vi "lightsheetMain.vi"() -> ()   [LabVIEW 2015]
panel:
  out "initLasers":T1(array[cluster])=[{"Component ID"="405nm", "COM Port"="COM14", "Type "=enum."omicronLuxX", "init"=1, "Max power (mW)"=60.0}, {"Component ID"="488nm", "COM Port"="COM4", "Type "=enum."omicronLuxX", "init"=1, "Max power (mW)"=60.0}, {"Component ID"="561nm", "COM Port"="COM27", "Type "=enum."coherentObis", "init"=1, "Max power (mW)"=50.0}, {"Component ID"="642nm", "COM Port"="COM12", "Type "=enum."omicronLuxX", "init"=1, "Max power (mW)"=140.0}]
  out "acquisitionTime":u32
  out "opticalSectionThickness (um)":dbl=5.0
  out "acqLaserCOM":refnum<visa-resource-name>[](array[refnum])
  out "acqLaserOff":string[](array[string])
  out "acqLaserOn":string[](array[string])
  out "acqFW":u8[](array[numeric])
  out "Lat x inc (mm)":dbl=0.37273599999999996
  out "Lat y inc (mm)":dbl=0.37273599999999996
  out "no y steps":i32=1
  out "no colours":i32=1
  out "no z imgs (acq)":i32=1
  out "no x steps":i32=1
  out "stop live view":bool
  out "LH yLim (mm)":dbl
  out "RH yLim (mm)":dbl
  in  "Set RH yLim":bool
  in  "Set LH yLim":bool
  out "TH zLim (mm)":dbl
  in  "Set TH zLim":bool
  in  "acqLSFM_3":enum32{"Acquisition (hardware)"}(tab)
  out "Generating tiff stacks":bool
  out "Acquisition in progress":bool
  in  "convertDcimgToTifStacks":bool=TRUE
  in  "setupAcq":bool
  in  "testAcq":bool
  out "x1":dbl
  out "y1":dbl
  out "z1":dbl
  out "x2":dbl
  out "y2":dbl
  out "z2":dbl
  in  "no z steps":i32=1
  in  "% FOV overlap":i32=10
  in  "z inc (um)":dbl=1.0
  in  "642":bool=TRUE
  in  "561":bool=TRUE
  in  "405":bool=TRUE
  in  "488":bool=TRUE
  in  "beginAcq":bool
  in  "stopAcq":bool
  in  "end all comms and exit":bool
  in  "acquisitionMode":enum32{"stop/start  ", "cont."}(radio)
  out "z inc (mm)":dbl=0.01
  in  "Save acq vals":bool
  in  "Read acq vals":bool
  out "Filter wheel":cluster{"FW Handle":u32, "init?":i16}={"FW Handle"=428794912, "init?"=1}
  out "sCMOS":cluster{"init":i16, "sCMOS handle":u32}
  out "Z stage":T2={"System no."=2, "zIdx"=1, "zLim (mm)"=0.0, "0, 1"=0}
  out "XY stage":T3={"System no."=1, "xIdx"=1, "yIdx"=2, "xLim (mm)"=0.0, "yLim (mm)"=0.0, "0, 1"=0}
  in  "LSFM_3":T4(tab)=enum."lasers/filters"
  out "acqDelay (ms)":u32=10
  out "fine axial vel (mm/s)":dbl=10.0
  in  "set axial vel":bool
  in  "filename":string="testImg"
  in  "Index":i32
  in  "Down":bool
  in  "Up":bool
  in  "Left":bool
  in  "Right":bool
  in  "Backward":bool
  in  "Forward":bool
  in  "Axial stepsize (mm/um)":dbl=1.0
  in  "Lateral stepsize (mm/um)":dbl=1.0
  in  "Toggle coarse/fine":enum32{"Coarse (mm) ", "Fine (um) "}(radio)
  out "x (mm)":dbl
  out "y (mm)":dbl
  out "z (mm)":dbl
  in  "Snap img":bool
  in  "set init xy pos":bool
  in  "set fin xy pos":bool
  in  "set init z":bool
  in  "set fin z":bool
  in  "mov init xy":bool
  in  "mov init z":bool
  in  "mov fin xy":bool
  in  "mov fin z":bool
  in  "coarse axial vel (mm/s)":dbl=6.0
  in  "642 nm power (mW)":dbl(slide)=54.0 min=0.0 max=60.0 step=1.0 scale=0.0..140.0
  in  "561 nm power (mW)":dbl(slide)=8.0 min=0.0 max=60.0 step=1.0 scale=0.0..60.0
  in  "488 nm power (mW)":dbl(slide)=5.0 min=0.0 max=60.0 step=1.0 scale=0.0..60.0
  in  "405 nm power (mW)":dbl(slide)=5.0 min=0.0 max=60.0 step=1.0 scale=0.0..60.0
  in  "FW pos":u16(ring)=4 items=["460/36 [DAPI]"=1, "525/50 [FITC]"=2, "605/70 [Cy3]"=3, "665/LP [Cy5]"=4, "Empty-1"=5, "Empty-2"=6]
  in  "next":bool
  in  "prev":bool
  in  "642 nm ON":bool
  in  "642 nm OFF":bool
  in  "561 nm ON":bool
  in  "561 nm OFF":bool
  in  "488 nm ON":bool
  in  "488 nm OFF":bool
  in  "405 nm ON":bool
  in  "405 nm OFF":bool
  in  "405 filter":u8(ring)=1 items=["460/36 [DAPI]"=1, "525/50 [FITC]"=2, "605/70 [Cy3]"=3, "665/LP [Cy5]"=4, "Empty-1"=5, "Empty-2"=6]
  in  "488 filter":u8(ring)=2 items=["460/36 [DAPI]"=1, "525/50 [FITC]"=2, "605/70 [Cy3]"=3, "665/LP [Cy5]"=4, "Empty-1"=5, "Empty-2"=6]
  in  "561 filter":u8(ring)=3 items=["460/36 [DAPI]"=1, "525/50 [FITC]"=2, "605/70 [Cy3]"=3, "665/LP [Cy5]"=4, "Empty-1"=5, "Empty-2"=6]
  in  "642 filter":u8(ring)=4 items=["460/36 [DAPI]"=1, "525/50 [FITC]"=2, "605/70 [Cy3]"=3, "665/LP [Cy5]"=4, "Empty-1"=5, "Empty-2"=6]
  out "Acquiring?":bool
  in  "live stream":bool
  in  "Set exp. time":bool
  in  "Exposure time (s)":dbl=1.0
  in  "stop live stream":bool
  in  "View stream":bool=TRUE
  out "Img. pixel size":dbl=0.26
  out "No. of pix":u16=2048
  in  "pixel binning":u16(ring) items=["1x1"=1, "2x2"=2, "4x4"=4]
  in  "No. pix":u16=2048
  in  "scmos pixel size (um)":dbl=6.5 format="%#_13g"
  out "FOV (mm)":dbl=0.53248
  in  "sensorSize":dbl=13.312 format="%#_13g"
  in  "Mag":dbl=25.0 format="%#_13g"
  in  "z":bool
  in  "xy":bool
  in  "488nm":bool=TRUE
  in  "405nm":bool=TRUE
  in  "561nm":bool=TRUE
  in  "642nm":bool=TRUE
  in  "sCMOS":bool
  in  "FW":bool=TRUE
  out "Appended path":path=path "C:/Users/LSFM_2/Desktop/dataAcq_2705/bothIllAxis/4umBead0.tif"
  in  "Base path":path=path "C:/Users/sims01/Desktop/dataAcq"
  in  "dcimgToStack":bool
  in  "stageAccDelay (ms)":u32
  # "Stage limits"
  # "Positions"
  # "Step sizes"
  # "Currrent positions"
  # "Motion control"
  # "Move stages"
  # "lasers"
  # "filters"
  # "File setup"
  # "Hardware initialization"
  # "Microscope properties"
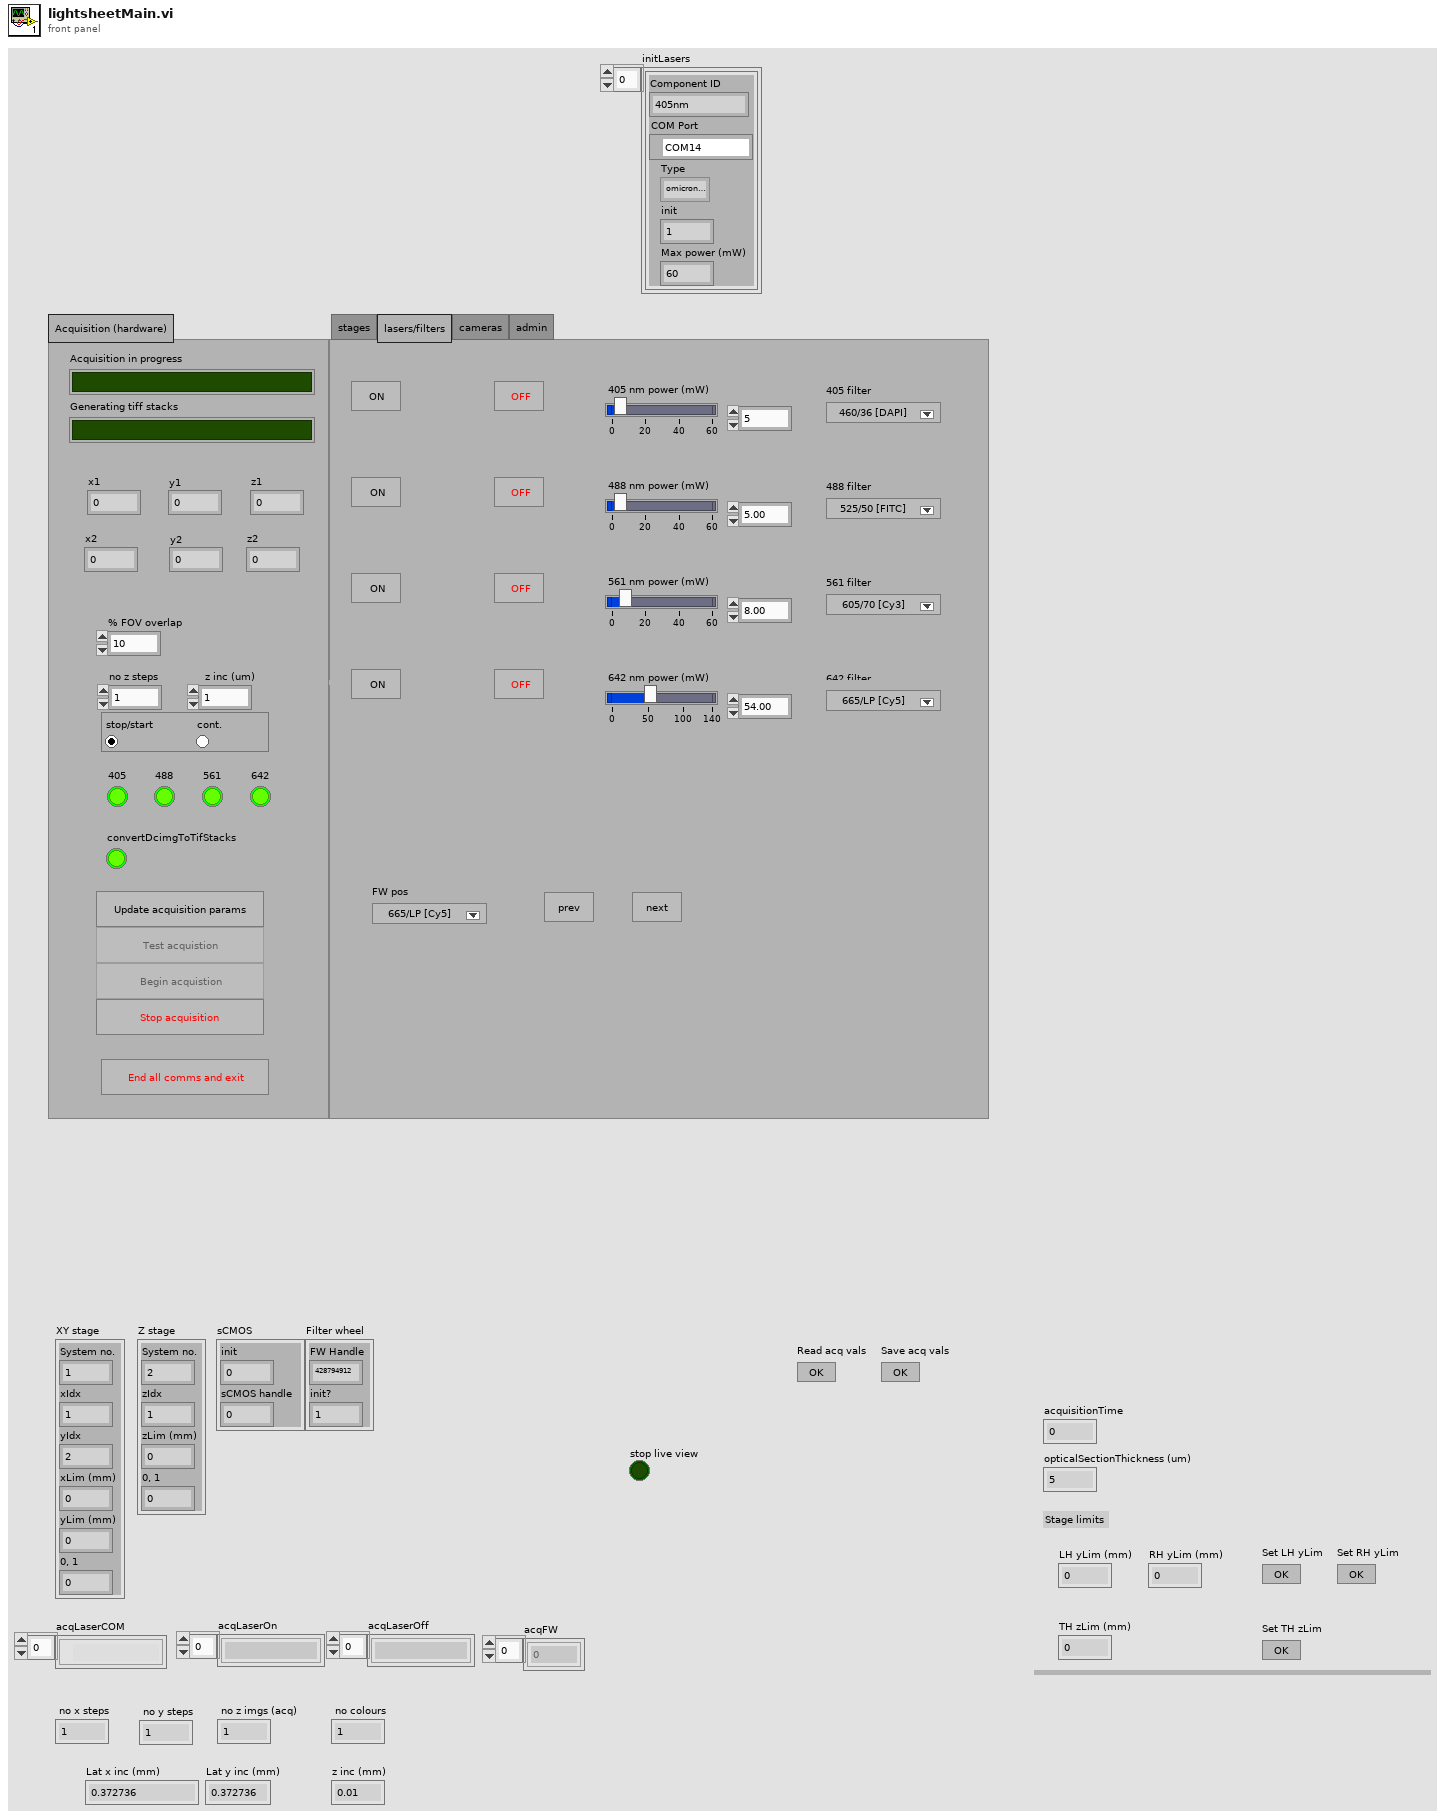
[diagram p1: front panel]
types:
  T1 = cluster{"Component ID":string, "COM Port":refnum<visa-resource-name>, "Type ":enum16{"omicronLuxX", "coherentObis"}, "init":i16, "Max power (mW)":dbl}[]
  T2 = cluster{"System no.":i32, "zIdx":i32, "zLim (mm)":dbl, "0, 1":i16}
  T3 = cluster{"System no.":i32, "xIdx":i32, "yIdx":i32, "xLim (mm)":dbl, "yLim (mm)":dbl, "0, 1":i16}
  T4 = enum32{"stages", "lasers/filters", "cameras", "admin"}
  T5 = enum8{"Enabled", "Disabled", "Disabled and Grayed Out"}
  T6 = cluster{"Component ID":string, "COM Port":refnum<visa-resource-name>, "Type ":enum16{"omicronLuxX", "coherentObis"}, "init":i16, "Max power (mW)":dbl}
  T7 = enum32{"Invalid", "Standard", "Closed", "Hidden", "Minimized", "Maximized"}
  T8 = cluster{"height":u32, "width":u32, "datatype":u32}
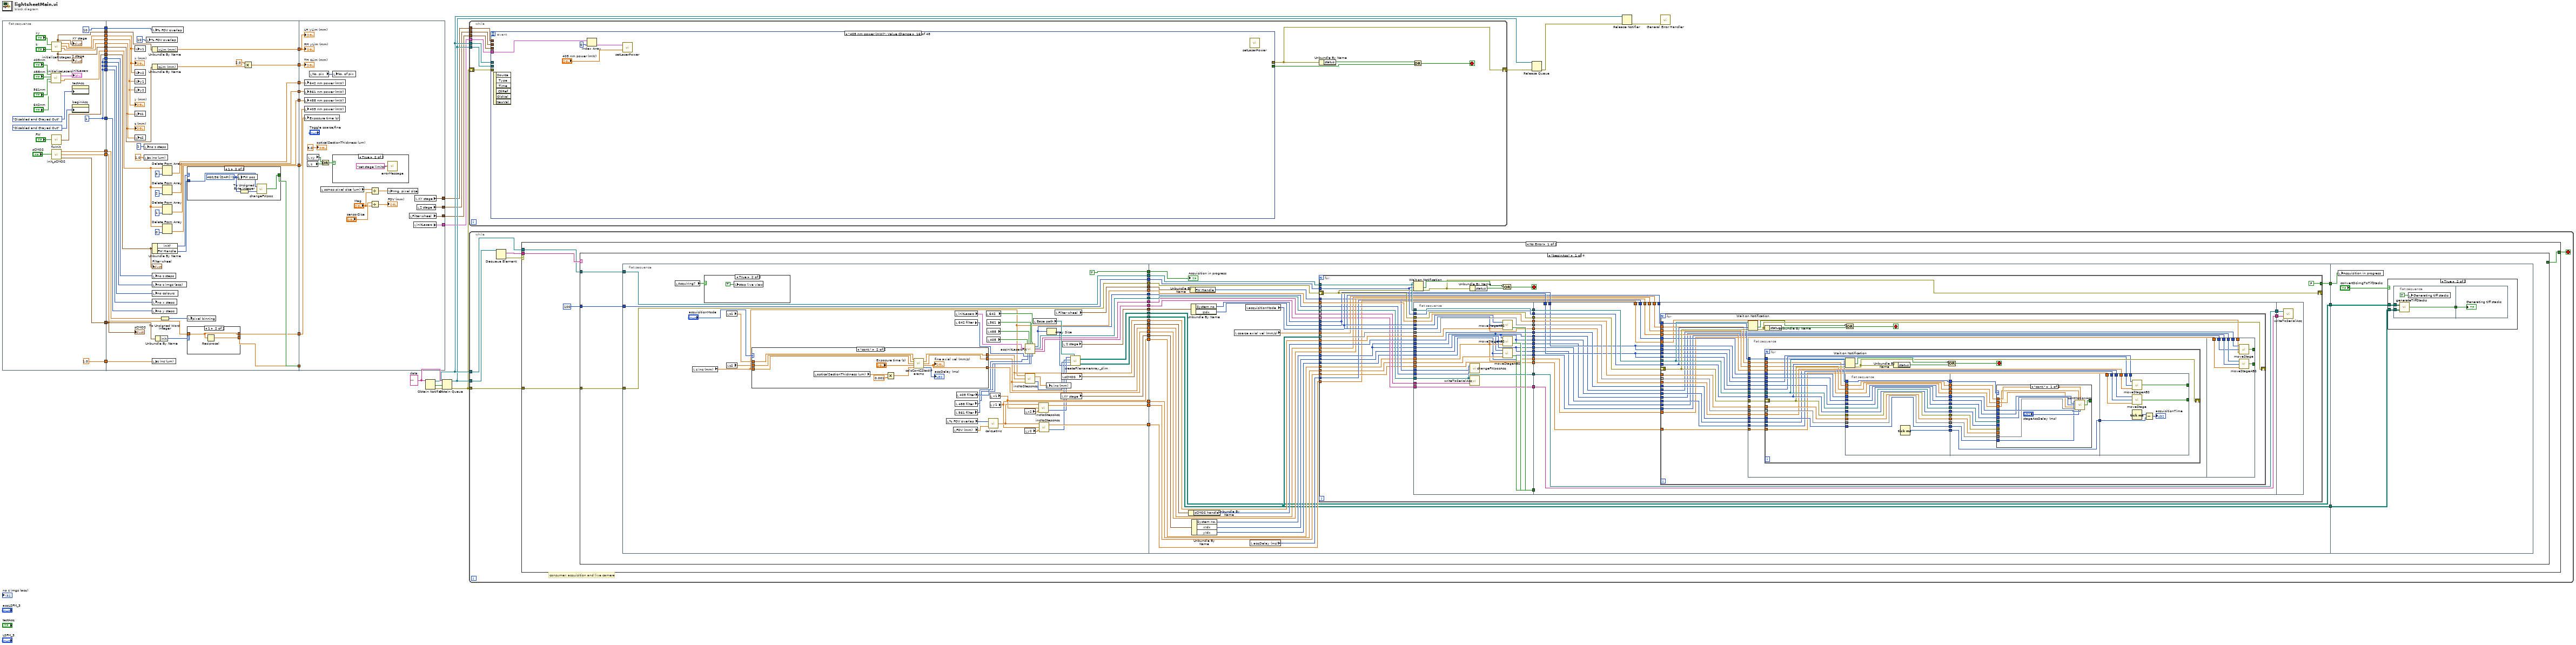
[diagram p0: block diagram]
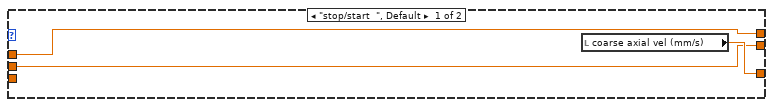
[diagram p3: hidden frame]
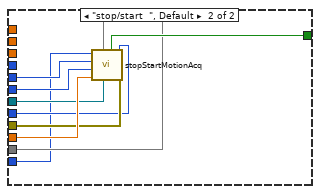
[diagram p4: hidden frame]
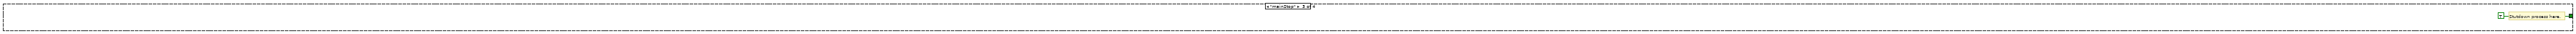
[diagram p7: hidden frame]
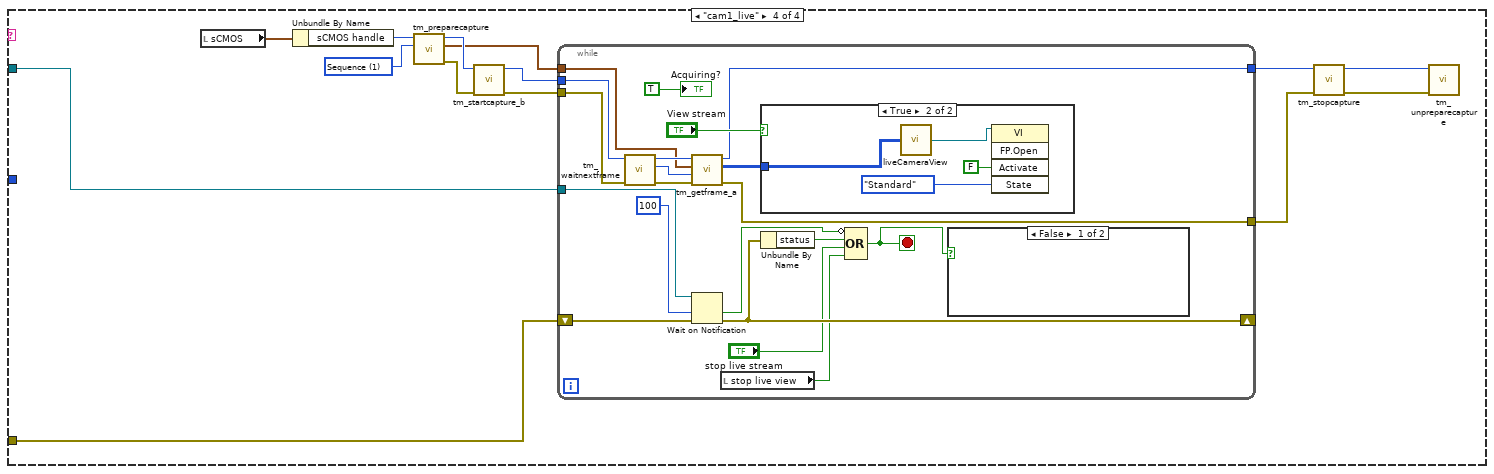
[diagram p8: hidden frame]
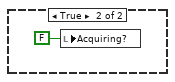
[diagram p9: hidden frame]
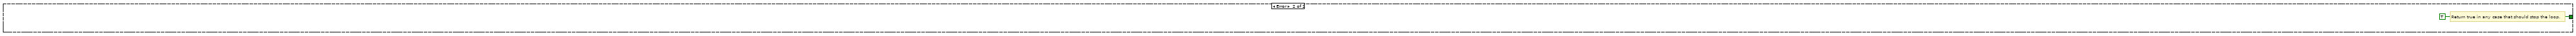
[diagram p11: hidden frame]
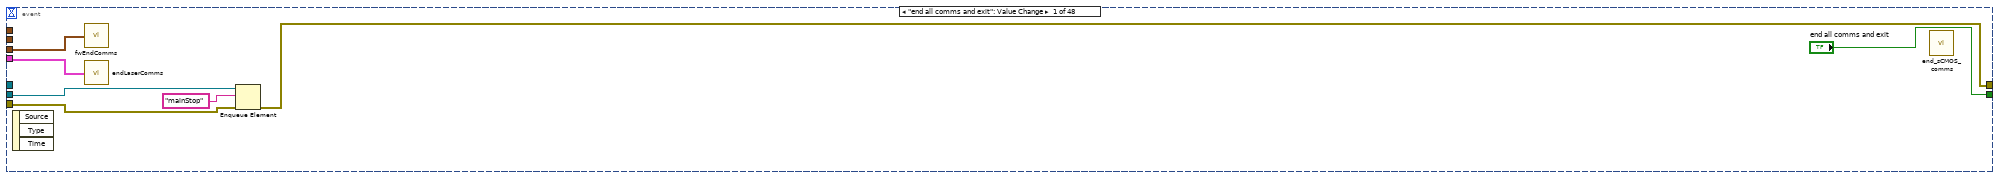
[diagram p12: hidden frame]
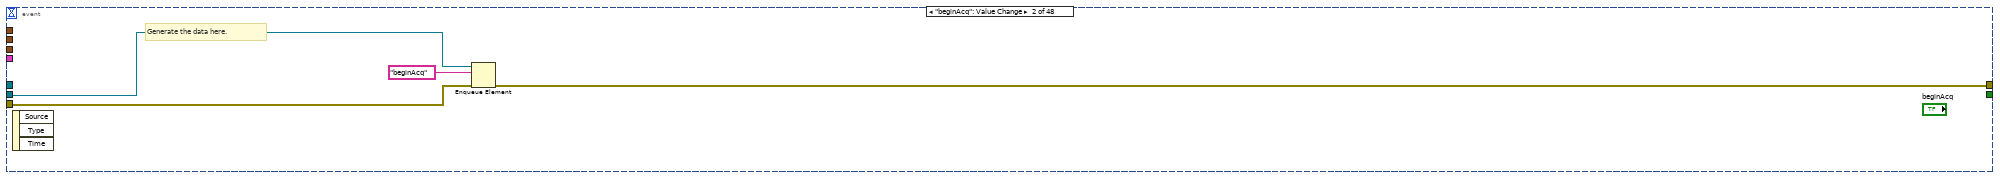
[diagram p13: hidden frame]
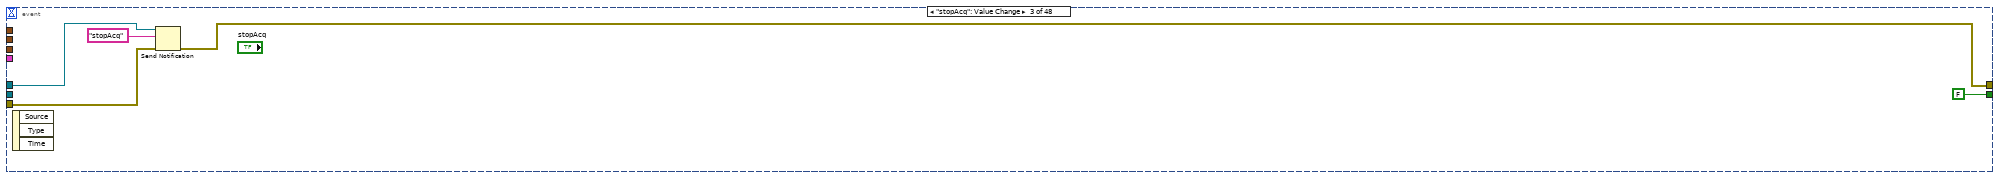
[diagram p14: hidden frame]
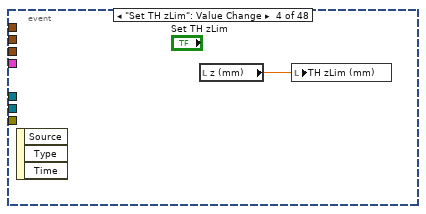
[diagram p15: hidden frame]
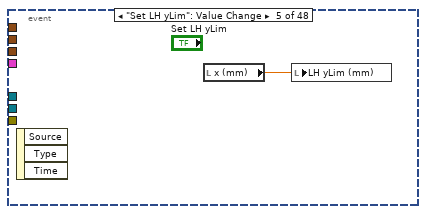
[diagram p16: hidden frame]
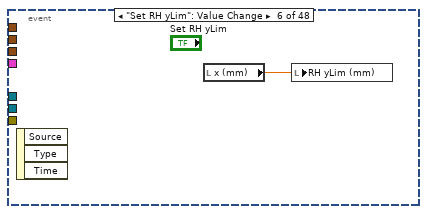
[diagram p17: hidden frame]
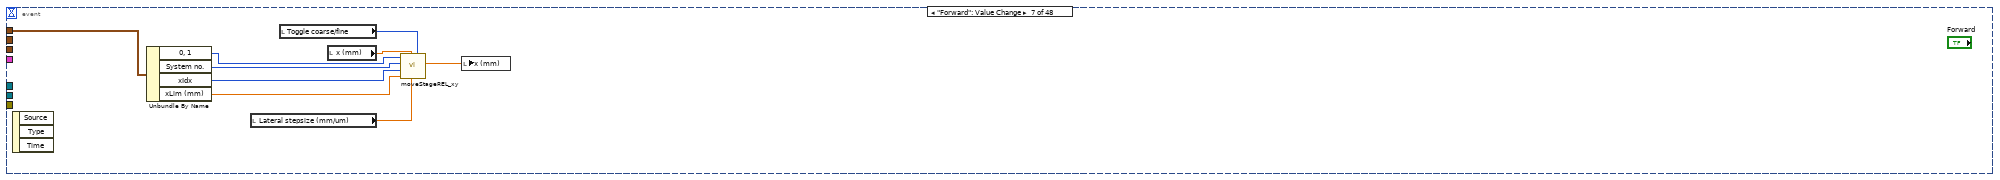
[diagram p18: hidden frame]
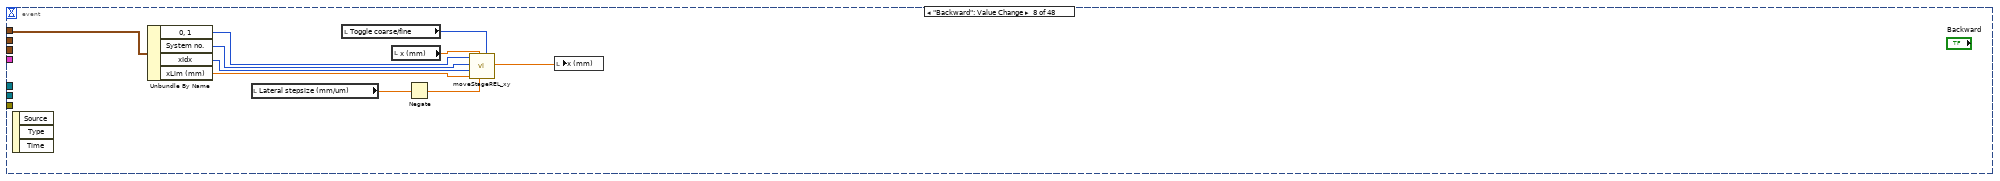
[diagram p19: hidden frame]
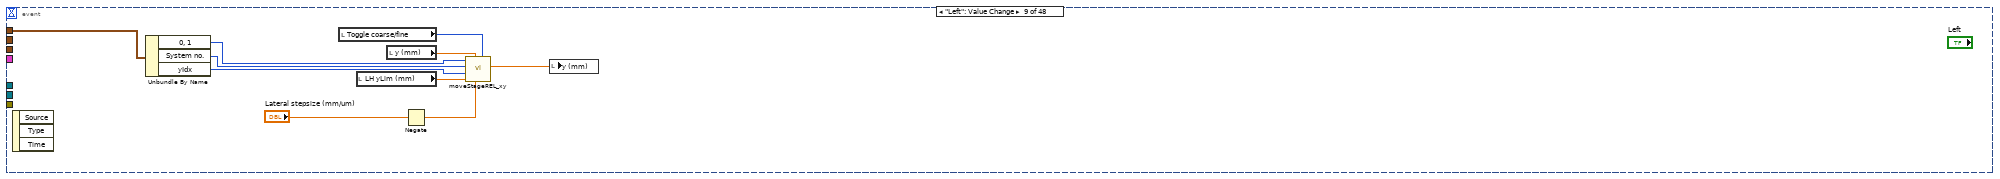
[diagram p20: hidden frame]
diagram:
  w28 = ""  # data
  n1 = flat-sequence {
    tunnel: [w61] -> w39
    tunnel: [w60] -> w38
    tunnel: [w59] -> w37
    tunnel: [w52] -> w36
    tunnel: [w51] -> w35
    tunnel: [w58] -> w34
    tunnel: [w57] -> w18
    tunnel: [w56] -> w17
    tunnel: [w50] -> w13
    tunnel: [w48] -> w12
    tunnel: [w48] -> w11
    tunnel: [w48] -> w10
    tunnel: [w48] -> w9
    tunnel: [10 ("% FOV overlap")] -> w8
    tunnel: [w48] -> w7
    tunnel: [1.0 ("z inc (um)")] -> w6
    tunnel: [w40] -> w5
    tunnel: w39 -> [w85]
    tunnel: w38 -> [w86]
    tunnel: w37 -> [w87]
    tunnel: w36 -> [w100]
    tunnel: w35 -> [w102]
    tunnel: w34 -> [w99]
    tunnel: [w96] -> w33
    tunnel: [w95] -> w32
    tunnel: [w94] -> w31
    tunnel: w18 -> [w93]
    tunnel: w17 -> [w92]
    tunnel: [w91] -> w16
    tunnel: [w90] -> w15
    tunnel: w13 -> [w81]
    tunnel: w12 -> [w80]
    tunnel: w11 -> [w79]
    tunnel: w10 -> [w78]
    tunnel: w9 -> [w77]
    tunnel: w8 -> [w76]
    tunnel: w7 -> [w75]
    tunnel: w6 -> [w74]
    tunnel: w5 -> [w65]
    tunnel: [w71] -> w4
    tunnel: [w69] -> w3
    tunnel: [w67] -> w2
    tunnel: [w64] -> w1
    tunnel: w33 -> [_]
    tunnel: w32 -> [w126]
    tunnel: w31 -> [_]
    tunnel: [w125] -> w20
    tunnel: [w124] -> w19
    tunnel: [w123] -> w21
    tunnel: w16 -> [w122]
    tunnel: w15 -> [w121]
    tunnel: [w115] -> w14
    tunnel: w4 -> [w114]
    tunnel: w3 -> [w113]
    tunnel: w2 -> [w112]
    tunnel: w1 -> [w111]
    frame #0 {
      w48 = 1 ("no y steps")
      n2 = call "initialiseLasers.vi"("642 nm"="642nm", "561 nm"="561nm", "488 nm"="488nm", "405 nm"="405nm") -> ("currLaserPowers"=w40:dbl[], "outputLasers"=→"initLasers":T1)
      n3 = call "fwInit.vi"("FW init?"="FW") -> ("Filter wheel init"=w58:cluster{"FW Handle":u32, "init?":i16})
      n4 = call "initializePIstages.vi"("xy stage"="xy", "z stage"="z") -> ("XY stage"=w56:T3, "Z stage"=w57:T2, "current xPos (mm)"=w61:dbl, "current yPos (mm)"=w60:dbl, "current zPos (mm)"=w59:dbl)  [unwired: 1 in]
      "XY stage" <- w56
      "Z stage" <- w57
      n5 = call "init_sCMOS.vi"("sCMOS_1"="sCMOS") -> ("Binning"=w50:dbl, "Exposure"=w52:dbl, "sCMOS init"=w51:cluster{"init":i16, "sCMOS handle":u32})
      n6 = property on="testAcq" class="Bool"("DisabledEnum"=T5."Disabled and Grayed Out" ("Disabled")) -> ()  [unwired: 2 in, 2 out]
      n7 = property on="beginAcq" class="Bool"("DisabledEnum"=T5."Disabled and Grayed Out" ("Disabled")) -> ()  [unwired: 2 in, 2 out]
    }
    frame #1 {
      n8 = local write "x1"(w85) -> ()
      n9 = local write "x2"(w85) -> ()
      n10 = local write "y1"(w86) -> ()
      n11 = local write "y2"(w86) -> ()
      n12 = local write "z1"(w87) -> ()
      n13 = local write "z2"(w87) -> ()
      n14 = local write "no z steps"(1 ("no z steps")) -> ()
      n15 = local write "z inc (um)"(1.0 ("z inc (um)")) -> ()
      n16 = local write "% FOV overlap"(10 ("% FOV overlap")) -> ()
      n17 = local write "% FOV overlap"(w76) -> ()
      n18 = Unbundle By Name(w92) -> ("xLim (mm)"=w91:dbl)
      n19 = Unbundle By Name(w93) -> ("zLim (mm)"=w89:dbl)
      n20 = Unbundle By Name(w99) -> ("init?"=w98:i16, "FW Handle"=w97:u32)
      n21 = local write "no z steps"(w75) -> ()
      n22 = local write "no z imgs (acq)"(w78) -> ()
      n23 = local write "no colours"(w79) -> ()
      n24 = local write "no x steps"(w77) -> ()
      n25 = local write "no y steps"(w80) -> ()
      n26 = local write "z inc (um)"(w74) -> ()
      n27 = Unbundle By Name(w102) -> ("init"=w101:i16)
      n28 = To Unsigned Word Integer(number=w81) -> (unsigned 16bit integer=w82:u16)
      n29 = Delete From Array(array=w65, index=3) -> (deleted portion=w64:dbl)  [unwired: 1 in, 1 out]
      n30 = Delete From Array(array=w65, index=2 ("length")) -> (deleted portion=w67:dbl)  [unwired: 1 in, 1 out]
      n31 = Delete From Array(array=w65, index=1 ("length")) -> (deleted portion=w69:dbl)  [unwired: 1 in, 1 out]
      n32 = Delete From Array(array=w65, index=0 ("length")) -> (deleted portion=w71:dbl)  [unwired: 1 in, 1 out]
      n33 = case shown="1" w98 {
        tunnel: w97 -> [_ w107]
        tunnel: [FALSE ("fwPosChanged") w106] -> w96
        frame 0, Default {
        }
        frame 1 {
          w104 = u16 1 items=["460/36 [DAPI]"=1, "525/50 [FITC]"=2, "605/70 [Cy3]"=3, "665/LP [Cy5]"=4, "Empty-1"=5, "Empty-2"=6] ("Filter wheel position")
          n34 = local write "FW pos"(w104) -> ()
          n35 = To Unsigned Byte Integer(number=w104) -> (unsigned 8bit integer=w105:u8)
          n36 = call "changeFWpos.vi"("FW pos"=w105, "FWhandle"=w107) -> ("fwPosChanged"=w106:bool)
        }
      }
      n37 = local write "pixel binning"(w82) -> ()
      n38 = case shown="1" w101 {
        tunnel: w100 -> [_ w110]
        tunnel: [w108 w110] -> w95
        tunnel: [w108 w109] -> w94
        frame 0, Default {
          w108 = 1.0
        }
        frame 1 {
          n39 = Reciprocal(x=w110) -> (1/x=w109:dbl)
        }
      }
      n40 = Multiply(x=2.0, y=w89) -> (x*y=w90:dbl)
      "z (mm)" <- w87
      "y (mm)" <- w86
      "x (mm)" <- w85
      "sCMOS" <- w102
      "Filter wheel" <- w99
    }
    frame #2 {
      n41 = local write "642 nm power (mW)"(w111) -> ()
      n42 = local write "561 nm power (mW)"(w112) -> ()
      n43 = local write "488 nm power (mW)"(w113) -> ()
      n44 = local write "405 nm power (mW)"(w114) -> ()
      n45 = local write "Exposure time (s)"(w126) -> ()
      n46 = local read "xy"() -> (w128:bool)
      n47 = local read "z"() -> (w127:bool)
      n48 = local read "No. pix"() -> (w117:u16)
      n49 = Or(x=w128, y=w127) -> (x .or. y?=w129:bool)
      n50 = local read "scmos pixel size (um)"() -> (w119:dbl)
      n51 = local write "No. of pix"(w117) -> ()
      n52 = case shown="True" w129 {
        frame False {
        }
        frame True {
          n53 = call "errorMessage.vi"("messageText"="set stage limits!") -> ()  [unwired: 3 out]
        }
      }
      n54 = Divide(x=w119, y="Mag") -> (x/y=w118:dbl)
      n55 = Divide(x="sensorSize", y="Mag") -> (x/y=→"FOV (mm)":dbl)
      n56 = local write "Img. pixel size"(w118) -> ()
      n57 = local read "Filter wheel"() -> (w125:cluster{"FW Handle":u32, "init?":i16})
      n58 = local read "initLasers"() -> (w115:T1)
      n59 = local read "XY stage"() -> (w124:T3)
      n60 = local read "Z stage"() -> (w123:T2)
      "TH zLim (mm)" <- w121
      "RH yLim (mm)" <- w122
      "LH yLim (mm)" <- w122
      "opticalSectionThickness (um)" <- 5.0 ("opticalSectionThickness (um)")
    }
  }
  n61 = Obtain Notifier(notification data type=w28) -> (notifier out=w24:refnum<notifier>, created new?=w30:bool, error out=w29:errorcluster)  [unwired: 3 in]
  n62 = Obtain Queue(element data type=w28, create if not found? (T)=w30, error in (no error)=w29) -> (queue out=w23:refnum<queue>, error out=w22:errorcluster)  [unwired: 2 in, 1 out]
  n63 = while {
    shift-right: [w139] -> w27
    shift-left: w22 -> [w142]
    tunnel: w23 -> [w143]
    tunnel: w24 -> [w137]
    tunnel: w21 -> [w136]
    tunnel: w20 -> [w135]
    tunnel: w19 -> [w134]
    tunnel: w14 -> [w133]
    stop <- w140 stop-if-true
    n64 = event shown="[15] \"405 nm power (mW)\": Value Change" {
      selector: _ -> [_ _ _ _ _ _ _ _ _ _ _ _ _ _ _ _ _ _ _ _ _ _ _ _ _ _ _ _ _ _ _ _ _ _ _ _ _ _ _ _ _ _ _ _ _ _ _ _]
      dyn-events: _ -> [_ _ _ _ _ _ _ _ _ _ _ _ _ _ _ _ _ _ _ _ _ _ _ _ _ _ _ _ _ _ _ _ _ _ _ _ _ _ _ _ _ _ _ _ _ _ _ _]
      timeout: _ -> [_ _ _ _ _ _ _ _ _ _ _ _ _ _ _ _ _ _ _ _ _ _ _ _ _ _ _ _ _ _ _ _ _ _ _ _ _ _ _ _ _ _ _ _ _ _ _ _]
      tunnel: w143 -> [w147 w154 _ _ _ _ _ _ _ _ _ _ _ _ _ _ _ _ _ _ _ _ _ _ _ _ _ _ _ w319 _ _ _ _ _ _ _ _ _ _ _ _ _ _ _ _ _ _]
      tunnel: w142 -> [w149 w153 w159 _ _ _ _ _ _ _ _ _ _ _ _ _ _ _ _ _ _ _ _ _ _ _ _ _ _ w321 _ _ _ _ _ _ _ _ _ _ _ _ _ _ _ _ _ _]
      tunnel: [w148 w152 w158 _ _ _ _ _ _ _ _ _ _ _ _ _ _ _ _ _ _ _ _ _ _ _ _ _ _ w320 _ _ _ _ _ _ _ _ _ _ _ _ _ _ _ _ _ _] -> w139
      tunnel: ["end all comms and exit" _ FALSE ("stop") _ _ _ _ _ _ _ _ _ _ _ _ _ _ _ _ _ _ _ _ _ _ _ _ _ _ _ _ _ _ _ _ _ _ _ _ _ _ _ _ _ _ _ _ _] -> w141
      tunnel: w137 -> [_ _ w157 _ _ _ _ _ _ _ _ _ _ _ _ _ _ _ _ _ _ _ _ _ _ _ _ _ _ _ _ _ _ _ _ _ _ _ _ _ _ _ _ _ _ _ _ _]
      tunnel: w136 -> [_ _ _ _ _ _ _ _ _ _ w209 w219 w221 _ _ _ _ _ _ _ _ _ _ _ _ _ _ _ _ _ _ _ _ _ _ _ _ _ _ w389 w393 _ _ _ _ _ w430 _]
      tunnel: w135 -> [w144 _ _ _ _ _ _ _ _ _ _ _ _ w224 _ _ w237 _ _ w253 _ _ w268 _ _ w284 w290 w301 _ _ _ _ _ _ _ _ _ _ _ _ _ _ _ _ _ _ w431 _]
      tunnel: w134 -> [_ _ _ _ _ _ w171 w181 w191 w200 _ _ _ _ _ _ _ _ _ _ _ _ _ _ _ _ _ _ _ _ _ _ _ _ _ w368 w369 _ _ _ _ _ _ _ _ _ w429 _]
      tunnel: w133 -> [w145 _ _ _ _ _ _ _ _ _ _ _ _ w226 w230 w235 w241 w245 w250 w256 w260 w265 w271 w275 w280 _ _ _ _ _ _ _ _ _ _ _ _ _ _ _ _ _ _ _ _ _ w427 _]
      event "end all comms and exit": Value Change {
        n65 = event-data() -> ()  [unwired: 1 in, 3 out]
        n66 = call "fwEndComms.vi"("fw cluster"=w144) -> ()
        n67 = call "endLaserComms.vi"("outputLasers"=w145) -> ()
        n68 = Enqueue Element(queue=w147, element="mainStop", error in (no error)=w149) -> (error out=w148:errorcluster)  [unwired: 1 in, 2 out]
        n69 = call "end_sCMOS_comms.vi"() -> ()  [unwired: 1 in]
      }
      event "beginAcq": Value Change {
        # "Generate the data here."
        n70 = event-data() -> ()  [unwired: 1 in, 3 out]
        n71 = Enqueue Element(queue=w154, element="beginAcq", error in (no error)=w153) -> (error out=w152:errorcluster)  [unwired: 1 in, 2 out]
      }
      event "stopAcq": Value Change {
        n72 = event-data() -> ()  [unwired: 1 in, 3 out]
        n73 = Send Notification(notification="stopAcq", notifier=w157, error in (no error)=w159) -> (error out=w158:errorcluster)  [unwired: 1 out]
      }
      event "Set TH zLim": Value Change {
        n74 = event-data() -> ()  [unwired: 1 in, 3 out]
        n75 = local read "z (mm)"() -> (w160:dbl)
        n76 = local write "TH zLim (mm)"(w160) -> ()
      }
      event "Set LH yLim": Value Change {
        n77 = event-data() -> ()  [unwired: 1 in, 3 out]
        n78 = local read "x (mm)"() -> (w161:dbl)
        n79 = local write "LH yLim (mm)"(w161) -> ()
      }
      event "Set RH yLim": Value Change {
        n80 = event-data() -> ()  [unwired: 1 in, 3 out]
        n81 = local read "x (mm)"() -> (w162:dbl)
        n82 = local write "RH yLim (mm)"(w162) -> ()
      }
      event "Forward": Value Change {
        n83 = event-data() -> ()  [unwired: 1 in, 3 out]
        n84 = Unbundle By Name(w171) -> ("0, 1"=w170:i16, "System no."=w169:i32, "xIdx"=w168:i32, "xLim (mm)"=w167:dbl)
        n85 = local read "Lateral stepsize (mm/um)"() -> (w166:dbl)
        n86 = local read "Toggle coarse/fine"() -> (w164:enum32{"Coarse (mm) ", "Fine (um) "})
        n87 = local read "x (mm)"() -> (w165:dbl)
        n88 = call "moveStageREL_xy.vi"("Radio Buttons"=w164, "increment"=w166, "initPos (mm)"=w165, "stage lim (mm)"=w167, "axisIdx"=w168, "System no."=w169, "stageInit"=w170) -> ("finPos"=w163:dbl)  [unwired: 3 in]
        n89 = local write "x (mm)"(w163) -> ()
      }
      event "Backward": Value Change {
        n90 = event-data() -> ()  [unwired: 1 in, 3 out]
        n91 = Unbundle By Name(w181) -> ("0, 1"=w180:i16, "System no."=w179:i32, "xIdx"=w178:i32, "xLim (mm)"=w177:dbl)
        n92 = local read "Lateral stepsize (mm/um)"() -> (w176:dbl)
        n93 = local read "Toggle coarse/fine"() -> (w174:enum32{"Coarse (mm) ", "Fine (um) "})
        n94 = local read "x (mm)"() -> (w173:dbl)
        n95 = Negate(x=w176) -> (-x=w175:dbl)
        n96 = call "moveStageREL_xy.vi"("Radio Buttons"=w174, "increment"=w175, "initPos (mm)"=w173, "stage lim (mm)"=w177, "axisIdx"=w178, "System no."=w179, "stageInit"=w180) -> ("finPos"=w172:dbl)  [unwired: 3 in]
        n97 = local write "x (mm)"(w172) -> ()
      }
      event "Left": Value Change {
        n98 = event-data() -> ()  [unwired: 1 in, 3 out]
        n99 = Unbundle By Name(w191) -> ("0, 1"=w189:i16, "System no."=w188:i32, "yIdx"=w187:i32)
        n100 = local read "Toggle coarse/fine"() -> (w184:enum32{"Coarse (mm) ", "Fine (um) "})
        n101 = local read "LH yLim (mm)"() -> (w186:dbl)
        n102 = local read "y (mm)"() -> (w183:dbl)
        n103 = Negate(x="Lateral stepsize (mm/um)") -> (-x=w185:dbl)
        n104 = call "moveStageREL_xy.vi"("Radio Buttons"=w184, "increment"=w185, "initPos (mm)"=w183, "stage lim (mm)"=w186, "axisIdx"=w187, "System no."=w188, "stageInit"=w189) -> ("finPos"=w182:dbl)  [unwired: 3 in]
        n105 = local write "y (mm)"(w182) -> ()
      }
      event "Right": Value Change {
        n106 = event-data() -> ()  [unwired: 1 in, 3 out]
        n107 = Unbundle By Name(w200) -> ("0, 1"=w198:i16, "System no."=w197:i32, "yIdx"=w196:i32)
        n108 = local read "Lateral stepsize (mm/um)"() -> (w193:dbl)
        n109 = local read "Toggle coarse/fine"() -> (w192:enum32{"Coarse (mm) ", "Fine (um) "})
        n110 = local read "RH yLim (mm)"() -> (w195:dbl)
        n111 = local read "y (mm)"() -> (w194:dbl)
        n112 = call "moveStageREL_xy.vi"("Radio Buttons"=w192, "increment"=w193, "initPos (mm)"=w194, "stage lim (mm)"=w195, "axisIdx"=w196, "System no."=w197, "stageInit"=w198) -> ("finPos"=w199:dbl)  [unwired: 3 in]
        n113 = local write "y (mm)"(w199) -> ()
      }
      event "Up": Value Change {
        n114 = event-data() -> ()  [unwired: 1 in, 4 out]
        n115 = Unbundle By Name(w209) -> ("0, 1"=w208:i16, "System no."=w207:i32, "zIdx"=w206:i32)
        n116 = local read "Toggle coarse/fine"() -> (w202:enum32{"Coarse (mm) ", "Fine (um) "})
        n117 = local read "TH zLim (mm)"() -> (w205:dbl)
        n118 = local read "z (mm)"() -> (w204:dbl)
        n119 = call "moveStageREL_z.vi"("Radio Buttons"=w202, "increment"="Axial stepsize (mm/um)", "initPos (mm)"=w204, "stage lim (mm)"=w205, "axisIdx"=w206, "System no."=w207, "stageInit"=w208) -> ("finPos"=w203:dbl)  [unwired: 3 in]
        n120 = local write "z (mm)"(w203) -> ()
      }
      event "Down": Value Change {
        n121 = event-data() -> ()  [unwired: 1 in, 4 out]
        n122 = Unbundle By Name(w219) -> ("0, 1"=w217:i16, "System no."=w216:i32, "zIdx"=w215:i32)
        n123 = local read "Axial stepsize (mm/um)"() -> (w218:dbl)
        n124 = local read "Toggle coarse/fine"() -> (w213:enum32{"Coarse (mm) ", "Fine (um) "})
        n125 = local read "TH zLim (mm)"() -> (w210:dbl)
        n126 = local read "z (mm)"() -> (w212:dbl)
        n127 = Negate(x=w218) -> (-x=w214:dbl)
        n128 = call "moveStageREL_z.vi"("Radio Buttons"=w213, "increment"=w214, "initPos (mm)"=w212, "stage lim (mm)"=w210, "axisIdx"=w215, "System no."=w216, "stageInit"=w217) -> ("finPos"=w211:dbl)  [unwired: 3 in]
        n129 = local write "z (mm)"(w211) -> ()
      }
      event "set axial vel": Value Change {
        n130 = event-data() -> ()  [unwired: 1 in, 6 out]
        n131 = call "setVel.vi"("vel (mm/s)"="coarse axial vel (mm/s)", "input cluster"=w221) -> ()
      }
      event "405 nm ON": Value Change {
        n132 = event-data() -> ()  [unwired: 1 in, 6 out]
        n133 = Index Array(array=w226, index=0) -> (element=w225:T6)
        n134 = call "changeLaserFW.vi"("FW pos"="405 filter", "inputFW"=w224, "inputLaser"=w225) -> ("changePos?"=w223:i16)
        n135 = case shown="0, Default" w223 {
          tunnel: "405 filter" -> [_ w229]
          frame 0, Default {
          }
          frame 1 {
            n136 = To Unsigned Word Integer(number=w229) -> (unsigned 16bit integer=w228:u16)
            n137 = local write "FW pos"(w228) -> ()
          }
        }
      }
      event "405 nm OFF": Value Change {
        n138 = event-data() -> ()  [unwired: 1 in, 6 out]
        n139 = Index Array(array=w230, index=0) -> (element=w232:T6)
        n140 = call "turnLaserOff.vi"("input cluster"=w232) -> ()  [unwired: 1 out]
      }
      event "405 nm power (mW)": Value Change {
        n141 = event-data() -> ()  [unwired: 1 in, 6 out]
        n142 = Index Array(array=w235, index=0) -> (element=w234:T6)
        n143 = call "setLaserPower.vi"("laser power (mW)"="405 nm power (mW)", "laser"=w234) -> ()  [unwired: 1 out]
        n144 = call "setLaserPower.vi"() -> ()  [unwired: 2 in, 1 out]
      }
      event "488 nm ON": Value Change {
        n145 = event-data() -> ()  [unwired: 1 in, 6 out]
        n146 = Index Array(array=w241, index=1) -> (element=w239:T6)
        n147 = call "changeLaserFW.vi"("FW pos"="488 filter", "inputFW"=w237, "inputLaser"=w239) -> ("changePos?"=w240:i16)
        n148 = case shown="0, Default" w240 {
          tunnel: "488 filter" -> [_ w244]
          frame 0, Default {
          }
          frame 1 {
            n149 = To Unsigned Word Integer(number=w244) -> (unsigned 16bit integer=w243:u16)
            n150 = local write "FW pos"(w243) -> ()
          }
        }
      }
      event "488 nm OFF": Value Change {
        n151 = event-data() -> ()  [unwired: 1 in, 6 out]
        n152 = Index Array(array=w245, index=1) -> (element=w246:T6)
        n153 = call "turnLaserOff.vi"("input cluster"=w246) -> ()  [unwired: 1 out]
      }
      event "488 nm power (mW)": Value Change {
        n154 = event-data() -> ()  [unwired: 1 in, 6 out]
        n155 = Index Array(array=w250, index=1) -> (element=w249:T6)
        n156 = call "setLaserPower.vi"("laser power (mW)"="488 nm power (mW)", "laser"=w249) -> ()  [unwired: 1 out]
      }
      event "561 nm ON": Value Change {
        n157 = event-data() -> ()  [unwired: 1 in, 6 out]
        n158 = Index Array(array=w256, index=2) -> (element=w254:T6)
        n159 = call "changeLaserFW.vi"("FW pos"="561 filter", "inputFW"=w253, "inputLaser"=w254) -> ("changePos?"=w255:i16)
        n160 = case shown="0, Default" w255 {
          tunnel: "561 filter" -> [_ w259]
          frame 0, Default {
          }
          frame 1 {
            n161 = To Unsigned Word Integer(number=w259) -> (unsigned 16bit integer=w258:u16)
            n162 = local write "FW pos"(w258) -> ()
          }
        }
      }
      event "561 nm OFF": Value Change {
        n163 = event-data() -> ()  [unwired: 1 in, 6 out]
        n164 = Index Array(array=w260, index=2) -> (element=w261:T6)
        n165 = call "turnLaserOff.vi"("input cluster"=w261) -> ()  [unwired: 1 out]
      }
      event "561 nm power (mW)": Value Change {
        n166 = event-data() -> ()  [unwired: 1 in, 6 out]
        n167 = Index Array(array=w265, index=2) -> (element=w264:T6)
        n168 = call "setLaserPower.vi"("laser power (mW)"="561 nm power (mW)", "laser"=w264) -> ()  [unwired: 1 out]
      }
      event "642 nm ON": Value Change {
        n169 = event-data() -> ()  [unwired: 1 in, 6 out]
        n170 = Index Array(array=w271, index=3) -> (element=w269:T6)
        n171 = call "changeLaserFW.vi"("FW pos"="642 filter", "inputFW"=w268, "inputLaser"=w269) -> ("changePos?"=w270:i16)
        n172 = case shown="0, Default" w270 {
          tunnel: "642 filter" -> [_ w274]
          frame 0, Default {
          }
          frame 1 {
            n173 = To Unsigned Word Integer(number=w274) -> (unsigned 16bit integer=w273:u16)
            n174 = local write "FW pos"(w273) -> ()
          }
        }
      }
      event "642 nm OFF": Value Change {
        n175 = event-data() -> ()  [unwired: 1 in, 6 out]
        n176 = Index Array(array=w275, index=3) -> (element=w276:T6)
        n177 = call "turnLaserOff.vi"("input cluster"=w276) -> ()  [unwired: 1 out]
      }
      event "642 nm power (mW)": Value Change {
        n178 = event-data() -> ()  [unwired: 1 in, 6 out]
        n179 = Index Array(array=w280, index=3) -> (element=w279:T6)
        n180 = call "setLaserPower.vi"("laser power (mW)"="642 nm power (mW)", "laser"=w279) -> ()  [unwired: 1 out]
      }
      event "FW pos": Value Change {
        n181 = event-data() -> ()  [unwired: 1 in, 6 out]
        n182 = Unbundle By Name(w284) -> ("init?"=w283:i16, "FW Handle"=w282:u32)
        n183 = case shown="1" w283 {
          tunnel: w282 -> [_ w289]
          tunnel: [FALSE w286] -> _
          frame 0, Default {
          }
          frame 1 {
            n184 = local read "FW pos"() -> (w288:u16)
            n185 = To Unsigned Byte Integer(number=w288) -> (unsigned 8bit integer=w287:u8)
            n186 = call "changeFWpos.vi"("FW pos"=w287, "FWhandle"=w289) -> ("fwPosChanged"=w286:bool)
          }
        }
      }
      event "prev": Value Change {
        n187 = event-data() -> ()  [unwired: 1 in, 6 out]
        n188 = Unbundle By Name(w290) -> ("init?"=w292:i16, "FW Handle"=w291:u32)
        n189 = case shown="0, Default" w292 {
          tunnel: w291 -> [_ w294]
          frame 0, Default {
          }
          frame 1 {
            n190 = local read "FW pos"() -> (w295:u16)
            n191 = case shown="2..6" w295 {
              tunnel: w295 -> [w298 _ w300]
              tunnel: [w297 u16 6 w300] -> w293
              frame 2..6 {
                n192 = Decrement(x=w298) -> (x-1=w297:u16)
              }
              frame 1 {
              }
              frame Default {
              }
            }
            n193 = local write "FW pos"(w293) -> ()
            n194 = To Unsigned Byte Integer(number=w293) -> (unsigned 8bit integer=w296:u8)
            n195 = call "changeFWpos.vi"("FW pos"=w296, "FWhandle"=w294) -> ()  [unwired: 1 out]
          }
        }
      }
      event "next": Value Change {
        n196 = event-data() -> ()  [unwired: 1 in, 6 out]
        n197 = Unbundle By Name(w301) -> ("init?"=w303:i16, "FW Handle"=w302:u32)
        n198 = case shown="1" w303 {
          tunnel: w302 -> [_ w305]
          frame 0, Default {
          }
          frame 1 {
            n199 = local read "FW pos"() -> (w306:u16)
            n200 = case shown="1..5" w306 {
              tunnel: w306 -> [w309 _ w311]
              tunnel: [w308 u16 1 w311] -> w304
              frame 1..5 {
                n201 = Increment(x=w309) -> (x+1=w308:u16)
              }
              frame 6 {
              }
              frame Default {
              }
            }
            n202 = local write "FW pos"(w304) -> ()
            n203 = To Unsigned Byte Integer(number=w304) -> (unsigned 8bit integer=w307:u8)
            n204 = call "changeFWpos.vi"("FW pos"=w307, "FWhandle"=w305) -> ()  [unwired: 1 out]
          }
        }
      }
      event "sCMOS": Value Change {
        n205 = event-data() -> ()  [unwired: 1 in, 6 out]
        n206 = call "init_sCMOS.vi"("sCMOS_1"=TRUE) -> ("Binning"=w314:dbl, "Exposure"=w313:dbl, "sCMOS init"=w316:cluster{"init":i16, "sCMOS handle":u32})
        n207 = local write "Exposure time (s)"(w313) -> ()
        n208 = local write "sCMOS"(w316) -> ()
        n209 = To Unsigned Word Integer(number=w314) -> (unsigned 16bit integer=w315:u16)
        n210 = local write "pixel binning"(w315) -> ()
      }
      event "live stream": Value Change {
        n211 = event-data() -> ()  [unwired: 1 in, 6 out]
        n212 = local read "sCMOS"() -> (w318:cluster{"init":i16, "sCMOS handle":u32})
        n213 = Unbundle By Name(w318) -> ("init"=w317:i16)
        n214 = case shown="0, Default" w317 {
          tunnel: w321 -> [w322 w325]
          tunnel: [w322 w324] -> w320
          tunnel: w319 -> [_ w323]
          frame 0, Default {
          }
          frame 1 {
            n215 = Enqueue Element(queue=w323, element="cam1_live", error in (no error)=w325) -> (error out=w324:errorcluster)  [unwired: 1 in, 2 out]
          }
        }
      }
      event "Set exp. time": Value Change {
        n216 = event-data() -> ()  [unwired: 1 in, 6 out]
        n217 = local read "Exposure time (s)"() -> (w328:dbl)
        n218 = local read "sCMOS"() -> (w327:cluster{"init":i16, "sCMOS handle":u32})
        n219 = call "setExposureTime.vi"("sCMOS cluster"=w327, "Exposure time (s)"=w328) -> ()
      }
      event "Snap img": Value Change {
        n220 = event-data() -> ()  [unwired: 1 in, 6 out]
        n221 = local read "sCMOS"() -> (w329:cluster{"init":i16, "sCMOS handle":u32})
        n222 = call "snapImgFULL.vi"("Index"="Index", "filename"="filename", "Base path"="Base path", "sCMOS cluster"=w329) -> ("Full file"=→"Appended path":path)
        n223 = Increment(x="Index") -> (x+1=w331:i32)
        n224 = local write "Index"(w331) -> ()
      }
      event "pixel binning": Value Change {
        n225 = event-data() -> ()  [unwired: 1 in, 6 out]
        n226 = local read "sCMOS"() -> (w335:cluster{"init":i16, "sCMOS handle":u32})
        n227 = call "binPixels.vi"("pixel binning"="pixel binning", "sCMOS cluster"=w335) -> ()
        n228 = To Double Precision Float(number="No. pix") -> (double precision float=w342:dbl)
        n229 = To Double Precision Float(number="pixel binning") -> (double precision float=w340:dbl)
        n230 = Multiply(x=w340, y="scmos pixel size (um)") -> (x*y=w338:dbl)
        n231 = Divide(x=w342, y=w340) -> (x/y=w345:dbl)
        n232 = local read "Mag"() -> (w337:dbl)
        n233 = To Unsigned Word Integer(number=w345) -> (unsigned 16bit integer=→"No. of pix":u16)
        n234 = Divide(x=w338, y=w337) -> (x/y=→"Img. pixel size":dbl)
      }
      event "set init xy pos": Value Change {
        n235 = event-data() -> ()  [unwired: 1 in, 6 out]
        n236 = local read "y (mm)"() -> (w354:dbl)
        "y1" <- w354
        n237 = local read "x (mm)"() -> (w346:dbl)
        "x1" <- w346
        n238 = local read "Lat y inc (mm)"() -> (w355:dbl)
        n239 = local read "Lat x inc (mm)"() -> (w348:dbl)
        n240 = local read "y2"() -> (w353:dbl)
        n241 = local read "x2"() -> (w347:dbl)
        n242 = call "incNoStepsAcq.vi"("finPos"=w347, "initPos"=w346, "inp inc (mm)"=w348) -> ("no steps"=w349:i32, "out inc (mm)"=w352:dbl)
        n243 = call "incNoStepsAcq.vi"("finPos"=w353, "initPos"=w354, "inp inc (mm)"=w355) -> ("no steps"=w350:i32, "out inc (mm)"=w351:dbl)
        n244 = local write "Lat y inc (mm)"(w351) -> ()
        n245 = local write "no y steps"(w350) -> ()
        n246 = local write "Lat x inc (mm)"(w352) -> ()
        n247 = local write "no x steps"(w349) -> ()
      }
      event "set fin xy pos": Value Change {
        n248 = event-data() -> ()  [unwired: 1 in, 6 out]
        n249 = local read "Lat y inc (mm)"() -> (w362:dbl)
        n250 = local read "Lat x inc (mm)"() -> (w365:dbl)
        n251 = local read "x (mm)"() -> (w363:dbl)
        "x2" <- w363
        n252 = local read "y (mm)"() -> (w360:dbl)
        "y2" <- w360
        n253 = local read "y1"() -> (w361:dbl)
        n254 = local read "x1"() -> (w364:dbl)
        n255 = call "incNoStepsAcq.vi"("finPos"=w363, "initPos"=w364, "inp inc (mm)"=w365) -> ("no steps"=w358:i32, "out inc (mm)"=w359:dbl)
        n256 = call "incNoStepsAcq.vi"("finPos"=w360, "initPos"=w361, "inp inc (mm)"=w362) -> ("no steps"=w356:i32, "out inc (mm)"=w357:dbl)
        n257 = local write "Lat x inc (mm)"(w359) -> ()
        n258 = local write "no x steps"(w358) -> ()
        n259 = local write "Lat y inc (mm)"(w357) -> ()
        n260 = local write "no y steps"(w356) -> ()
      }
      event "mov init xy": Value Change {
        n261 = event-data() -> ()  [unwired: 1 in, 6 out]
        n262 = local read "x1"() -> (w366:dbl)
        n263 = local read "y1"() -> (w367:dbl)
        n264 = call "movXY.vi"("y pos (mm)"=w367, "x pos (mm)"=w366, "xy cluster"=w368) -> ()
      }
      event "mov fin xy": Value Change {
        n265 = event-data() -> ()  [unwired: 1 in, 6 out]
        n266 = local read "x2"() -> (w370:dbl)
        n267 = local read "y2"() -> (w371:dbl)
        n268 = call "movXY.vi"("y pos (mm)"=w371, "x pos (mm)"=w370, "xy cluster"=w369) -> ()
      }
      event "set init z": Value Change {
        n269 = event-data() -> ()  [unwired: 1 in, 6 out]
        n270 = local read "z (mm)"() -> (w374:dbl)
        "z1" <- w374
        n271 = local read "z inc (mm)"() -> (w376:dbl)
        n272 = local read "z2"() -> (w375:dbl)
        n273 = call "incNoStepsAcq.vi"("finPos"=w375, "initPos"=w374, "inp inc (mm)"=w376) -> ("no steps"=w373:i32, "out inc (mm)"=w372:dbl)
        n274 = local write "z inc (mm)"(w372) -> ()
        n275 = local write "no z imgs (acq)"(w373) -> ()
        n276 = local write "no z steps"(w373) -> ()
        n277 = call "mmToUm.vi"("distance (mm)"=w372) -> ("distance (um)"=w378:dbl)
        n278 = Absolute Value(x=w378) -> (abs(x)=w377:dbl)
        n279 = local write "z inc (um)"(w377) -> ()
      }
      event "set fin z": Value Change {
        n280 = event-data() -> ()  [unwired: 1 in, 6 out]
        n281 = local read "z inc (mm)"() -> (w383:dbl)
        n282 = local read "z (mm)"() -> (w381:dbl)
        "z2" <- w381
        n283 = local read "z1"() -> (w382:dbl)
        n284 = call "incNoStepsAcq.vi"("finPos"=w381, "initPos"=w382, "inp inc (mm)"=w383) -> ("no steps"=w380:i32, "out inc (mm)"=w379:dbl)
        n285 = local write "z inc (mm)"(w379) -> ()
        n286 = local write "no z imgs (acq)"(w380) -> ()
        n287 = local write "no z steps"(w380) -> ()
        n288 = call "mmToUm.vi"("distance (mm)"=w379) -> ("distance (um)"=w385:dbl)
        n289 = Absolute Value(x=w385) -> (abs(x)=w384:dbl)
        n290 = local write "z inc (um)"(w384) -> ()
      }
      event "mov init z": Value Change {
        n291 = event-data() -> ()  [unwired: 1 in, 6 out]
        n292 = Unbundle By Name(w389) -> ("System no."=w388:i32, "zIdx"=w387:i32)
        n293 = local read "z1"() -> (w386:dbl)
        n294 = call "moveStageABS.vi"("absolute pos (mm)"=w386, "axisIdx"=w387, "System no."=w388) -> ()  [unwired: 1 out]
      }
      event "mov fin z": Value Change {
        n295 = event-data() -> ()  [unwired: 1 in, 6 out]
        n296 = Unbundle By Name(w393) -> ("System no."=w392:i32, "zIdx"=w391:i32)
        n297 = local read "z2"() -> (w390:dbl)
        n298 = call "moveStageABS.vi"("absolute pos (mm)"=w390, "axisIdx"=w391, "System no."=w392) -> ()  [unwired: 1 out]
      }
      event "Read acq vals": Value Change {
        n299 = event-data() -> ()  [unwired: 1 in, 6 out]
      }
      event "Save acq vals": Value Change {
        n300 = event-data() -> ()  [unwired: 1 in, 6 out]
      }
      event "z inc (um)": Value Change {
        n301 = event-data() -> ()  [unwired: 1 in, 6 out]
        n302 = call "umTomm.vi"("distance (um)"="z inc (um)") -> ("distance (mm)"=w398:dbl)
        n303 = local read "z1"() -> (w397:dbl)
        n304 = local read "z2"() -> (w396:dbl)
        n305 = call "incNoStepsAcq.vi"("finPos"=w396, "initPos"=w397, "inp inc (mm)"=w398) -> ("no steps"=w394:i32, "out inc (mm)"=w395:dbl)
        n306 = local write "z inc (mm)"(w395) -> ()
        n307 = local write "no z steps"(w394) -> ()
        n308 = local write "no z imgs (acq)"(w394) -> ()
      }
      event "no z steps": Value Change {
        n309 = event-data() -> ()  [unwired: 1 in, 6 out]
        n310 = local read "z2"() -> (w403:dbl)
        n311 = local read "z1"() -> (w404:dbl)
        n312 = local write "no z imgs (acq)"("no z steps") -> ()
        n313 = call "calcInc.vi"("no. steps"="no z steps", "init pos (mm)"=w404, "fin pos (mm)"=w403) -> ("inc (mm)"=w401:dbl)
        n314 = local write "z inc (mm)"(w401) -> ()
        n315 = call "mmToUm.vi"("distance (mm)"=w401) -> ("distance (um)"=w405:dbl)
        n316 = Absolute Value(x=w405) -> (abs(x)=w402:dbl)
        n317 = local write "z inc (um)"(w402) -> ()
      }
      event "% FOV overlap": Value Change {
        n318 = event-data() -> ()  [unwired: 1 in, 6 out]
        n319 = local read "FOV (mm)"() -> (w415:dbl)
        n320 = call "calcLatInc.vi"("FOV (mm)"=w415, "% FOV overlap"="% FOV overlap") -> ("Lateral increment (mm)"=w409:dbl)
        n321 = local read "x1"() -> (w410:dbl)
        n322 = local read "x2"() -> (w408:dbl)
        n323 = local read "y1"() -> (w414:dbl)
        n324 = local read "y2"() -> (w413:dbl)
        n325 = call "incNoStepsAcq.vi"("finPos"=w408, "initPos"=w410, "inp inc (mm)"=w409) -> ("no steps"=→"no x steps":i32, "out inc (mm)"=→"Lat x inc (mm)":dbl)
        n326 = call "incNoStepsAcq.vi"("finPos"=w413, "initPos"=w414, "inp inc (mm)"=w409) -> ("no steps"=→"no y steps":i32, "out inc (mm)"=→"Lat y inc (mm)":dbl)
      }
      event "setupAcq": Value Change {
        n327 = event-data() -> ()  [unwired: 1 in, 6 out]
        n328 = local read "Acquiring?"() -> (w444:bool)
        n329 = local read "Base path"() -> (w426:path)
        n330 = local read "488 filter"() -> (w442:u8)
        n331 = local read "561 filter"() -> (w441:u8)
        n332 = local read "642 filter"() -> (w440:u8)
        n333 = local read "405 filter"() -> (w443:u8)
        n334 = Concatenate Strings("*" ("string"), "dcimg" ("string")) -> (w425:string)
        n335 = case shown="True" w444 {
          frame False {
          }
          frame True {
            "stop live view" <- TRUE ("stop live view")
          }
        }
        n336 = List Folder(path=w426, pattern=w425) -> (filenames=w422:string[])  [unwired: 2 in, 3 out]
        n337 = Array Size(array=w422) -> (size(s)=w419:i32)
        n338 = call "acqComponentsInit_v3.vi"("XY stage"=w429, "Z stage"=w430, "Filter wheel init"=w431, "LSFM_3 lasers"=w427, "405 nm (aq)"="405", "405 filter"=w443, "488 nm (aq)"="488", "488 filter"=w442, "561 nm (aq)"="561", "561 filter"=w441, "642 nm (aq)"="642", "642 filter"=w440) -> ("corrCompsInit?"=w420:i16, "noColours"=w428:i32, "FWpos"=→"acqFW":u8[], "acqLaserCOM"=→"acqLaserCOM":refnum<visa-resource-name>[], "acqLaserOff"=→"acqLaserOff":string[], "acqLaserOn"=→"acqLaserOn":string[])  [unwired: 2 in]
        "no colours" <- w428
        n339 = Equal To 0?(x=w419) -> (x = 0?=w418:bool)
        n340 = Boolean To (0,1)(Boolean=w418) -> (0, 1=w417:i16)
        n341 = case shown="0, Default" w417 {
          frame 0, Default {
            n342 = call "errorMessage.vi"("messageText"="There are already images in the specifed file.\nChange the specified file or delete these images.") -> ()  [unwired: 3 out]
          }
          frame 1 {
          }
        }
        n343 = And(x=w417, y=w420) -> (x .and. y?=w421:i16)
        n344 = case shown="1" w421 {
          tunnel: w428 -> [_ _]
          frame 0, Default {
            n345 = call "errorMessage.vi"("messageText"="One or more of the required components has not been intialized correctly.") -> ()  [unwired: 3 out]
          }
          frame 1 {
            n346 = local read "acquisitionMode"() -> (w447:enum32{"stop/start  ", "cont."})
            n347 = local read "% FOV overlap"() -> (w461:i32)
            n348 = local read "z inc (mm)"() -> (w448:dbl)
            n349 = local read "FOV (mm)"() -> (w460:dbl)
            n350 = property on="testAcq" class="Bool"("DisabledEnum"=T5."Enabled" ("Disabled")) -> ()  [unwired: 2 in, 2 out]
            n351 = property on="beginAcq" class="Bool"("DisabledEnum"=T5."Enabled" ("Disabled")) -> ()  [unwired: 2 in, 2 out]
            n352 = property on="stopAcq" class="Bool"("DisabledEnum"=T5."Enabled" ("Disabled")) -> ()  [unwired: 2 in, 2 out]
            n353 = call "calcLatInc.vi"("FOV (mm)"=w460, "% FOV overlap"=w461) -> ("Lateral increment (mm)"=w456:dbl)
            n354 = local read "z1"() -> (w450:dbl)
            n355 = local read "z2"() -> (w449:dbl)
            n356 = local read "x1"() -> (w457:dbl)
            n357 = local read "x2"() -> (w455:dbl)
            n358 = local read "y1"() -> (w459:dbl)
            n359 = local read "y2"() -> (w458:dbl)
            n360 = case shown="\"cont.\"" w447 {
              tunnel: w450 -> [_ w473]
              tunnel: w448 -> [_ w472]
              tunnel: w449 -> [_ w469]
              frame "stop/start  ", Default {
              }
              frame "cont." {
                n361 = local read "opticalSectionThickness (um)"() -> (w475:dbl)
                n362 = local read "Exposure time (s)"() -> (w471:dbl)
                n363 = Multiply(x=w475, y=0.001) -> (x*y=w470:dbl)
                n364 = call "calcContZStackParams.vi"("zPosInit (mm)"=w473, "zPosFin (mm)"=w469, "zIncrement (mm)"=w472, "Exposure time (s)"=w471, "opticalSectionThickness(mm)"=w470) -> ("new zPosInit (mm)"=w468:dbl, "new zPosFin (mm)"=w467:dbl, "fine axial vel (mm/s)"=w466:dbl, "acqDelay (ms)"=w465:u32)  [unwired: 7 in]
                n365 = local write "z1"(w468) -> ()
                n366 = local write "z2"(w467) -> ()
                n367 = local write "fine axial vel (mm/s)"(w466) -> ()
                n368 = local write "acqDelay (ms)"(w465) -> ()
              }
            }
            n369 = call "incNoStepsAcq.vi"("finPos"=w455, "initPos"=w457, "inp inc (mm)"=w456) -> ("no steps"=w452:i32, "out inc (mm)"=w454:dbl)
            n370 = call "incNoStepsAcq.vi"("finPos"=w458, "initPos"=w459, "inp inc (mm)"=w456) -> ("no steps"=w451:i32, "out inc (mm)"=w453:dbl)
            n371 = local write "Lat x inc (mm)"(w454) -> ()
            n372 = local write "no x steps"(w452) -> ()
            n373 = local write "Lat y inc (mm)"(w453) -> ()
            n374 = local write "no y steps"(w451) -> ()
          }
        }
      }
      event "dcimgToStack": Value Change {
        n375 = event-data() -> ()  [unwired: 1 in, 6 out]
        n376 = flat-sequence {
          tunnel: [TRUE ("Generating tiff stacks")] -> w478
          tunnel: [w483] -> w479
          tunnel: w478 -> [w482]
          tunnel: [FALSE ("Generating tiff stacks")] -> w477
          tunnel: w479 -> [_]
          tunnel: w477 -> [w486]
          frame #0 {
          }
          frame #1 {
            n377 = local write "Generating tiff stacks"(w482) -> ()
            n378 = local read "Base path"() -> (w484:path)
            n379 = call "convertDCIMGsInFileToTifStack.vi"("fileExtension"="dcimg", "path"=w484) -> ("stackConvComplete"=w483:bool)
          }
          frame #2 {
            n380 = local write "Generating tiff stacks"(w486) -> ()
          }
        }
      }
    }
    n381 = Unbundle By Name(w139) -> ("status"=w138:bool)
    n382 = Or(x=w138, y=w141) -> (x .or. y?=w140:bool)
  }
  n383 = while {
    tunnel: w23 -> [w492]
    tunnel: w24 -> [w488]
    tunnel: w22 -> [w487]
    stop <- w489 stop-if-true
    # "consumer: acquisition and live camera"
    n384 = Dequeue Element(queue=w492) -> (element=w490:string, error out=w491:errorcluster)  [unwired: 2 in, 2 out]
    n385 = case shown="No Error" w491 {
      tunnel: w490 -> [w497 _]
      tunnel: [w496 TRUE] -> w489
      tunnel: w488 -> [w495 _]
      tunnel: w487 -> [w494 _]
      frame No Error {
        n386 = case shown="\"beginAcq\"" w497 {
          tunnel: [_ _ TRUE _] -> w496
          tunnel: w495 -> [w525 _ _ w894]
          tunnel: w494 -> [w524 _ _ w893]
          tunnel: 100 ("timeout in ms (-1)") -> [w523 _ _ _]
          frame "beginAcq" {
            n387 = flat-sequence {
              tunnel: w523 -> [w569]
              tunnel: w524 -> [w570]
              tunnel: w525 -> [w571]
              tunnel: [w571] -> w522
              tunnel: [w570] -> w521
              tunnel: [w569] -> w520
              tunnel: [w537] -> w519
              tunnel: [w538] -> w518
              tunnel: [w567] -> w517
              tunnel: [w566] -> w516
              tunnel: [w564] -> w515
              tunnel: [w529] -> w514
              tunnel: [w535] -> w513
              tunnel: [w562] -> w512
              tunnel: [w534] -> w511
              tunnel: [w546] -> w510
              tunnel: [w545] -> w509
              tunnel: [w544] -> w508
              tunnel: [w543] -> w507
              tunnel: [w542] -> w506
              tunnel: [w541] -> w505
              tunnel: [w540] -> w504
              tunnel: [w539] -> w503
              tunnel: [TRUE ("Acquisition in progress")] -> w500
              tunnel: [w527] -> w498
              tunnel: w522 -> [w619]
              tunnel: w521 -> [w618]
              tunnel: w520 -> [w617]
              tunnel: w519 -> [w592]
              tunnel: w518 -> [w591]
              tunnel: w517 -> [w616]
              tunnel: w516 -> [w611]
              tunnel: w515 -> [w609]
              tunnel: w514 -> [w608]
              tunnel: w513 -> [w607]
              tunnel: w512 -> [w606]
              tunnel: w511 -> [w604]
              tunnel: w510 -> [w603]
              tunnel: w509 -> [w602]
              tunnel: w508 -> [w601]
              tunnel: w507 -> [w600]
              tunnel: w506 -> [w596]
              tunnel: w505 -> [w595]
              tunnel: w504 -> [w594]
              tunnel: w503 -> [w593]
              tunnel: [w592] -> w502
              tunnel: [w591] -> w501
              tunnel: w500 -> [w589]
              tunnel: [w588] -> w499
              tunnel: w498 -> [w587]
              tunnel: w502 -> [w876]
              tunnel: w501 -> [w877]
              tunnel: w499 -> [w879]
              frame #0 {
                n388 = local read "Acquiring?"() -> (w556:bool)
                n389 = local read "z inc (mm)"() -> (w535:dbl)
                n390 = case shown="True" w556 {
                  frame False {
                  }
                  frame True {
                    n391 = local write "stop live view"(TRUE ("stop live view")) -> ()
                  }
                }
                n392 = local read "z1"() -> (w563:dbl)
                n393 = local read "z2"() -> (w528:dbl)
                n394 = case shown="\"cont.\"" "acquisitionMode" {
                  tunnel: [w574 w579] -> w564
                  tunnel: [w575 w578] -> w529
                  tunnel: w563 -> [w575 w584]
                  tunnel: w535 -> [_ w583]
                  tunnel: w528 -> [w573 w581]
                  tunnel: [w573 w577] -> w527
                  frame "stop/start  ", Default {
                    n395 = local read "coarse axial vel (mm/s)"() -> (w574:dbl)
                  }
                  frame "cont." {
                    n396 = local read "opticalSectionThickness (um)"() -> (w586:dbl)
                    n397 = Multiply(x=w586, y=0.001) -> (x*y=w582:dbl)
                    n398 = call "calcContZStackParams.vi"("zPosInit (mm)"=w584, "zPosFin (mm)"=w581, "zIncrement (mm)"=w583, "Exposure time (s)"="Exposure time (s)", "opticalSectionThickness(mm)"=w582) -> ("new zPosInit (mm)"=w578:dbl, "new zPosFin (mm)"=w577:dbl, "fine axial vel (mm/s)"=w579:dbl, "acqDelay (ms)"=→"acqDelay (ms)":u32)  [unwired: 7 in]
                    "fine axial vel (mm/s)" <- w579
                  }
                }
                n399 = local read "% FOV overlap"() -> (w557:i32)
                n400 = local read "FOV (mm)"() -> (w558:dbl)
                n401 = local read "initLasers"() -> (w526:T1)
                n402 = local read "642 filter"() -> (w547:u8)
                n403 = local read "488 filter"() -> (w549:u8)
                n404 = local read "561 filter"() -> (w548:u8)
                n405 = local read "405 filter"() -> (w550:u8)
                n406 = local read "642"() -> (w553:bool)
                n407 = local read "561"() -> (w552:bool)
                n408 = local read "488"() -> (w551:bool)
                n409 = local read "405"() -> (w554:bool)
                n410 = call "calcLatInc.vi"("FOV (mm)"=w558, "% FOV overlap"=w557) -> ("Lateral increment (mm)"=w560:dbl)
                n411 = local read "x1"() -> (w542:dbl)
                n412 = local read "y1"() -> (w541:dbl)
                n413 = local read "x2"() -> (w561:dbl)
                n414 = local read "y2"() -> (w559:dbl)
                n415 = call "acqInitLasersFW.vi"("LSFM_3 lasers"=w526, "405 nm (aq)"=w554, "405 filter"=w550, "488 nm (aq)"=w551, "488 filter"=w549, "561 nm (aq)"=w552, "561 filter"=w548, "642 nm (aq)"=w553, "642 filter"=w547) -> ("FWpos"=w534:u8[], "acqLaserCOM"=w546:refnum<visa-resource-name>[], "acqLaserOn"=w545:string[], "acqLaserOff"=w544:string[])  [unwired: 7 in]
                n416 = call "incNoStepsAcq.vi"("finPos"=w527, "initPos"=w529, "inp inc (mm)"=w535) -> ("no steps"=w531:i32, "out inc (mm)"=w555:dbl)
                n417 = local read "Base path"() -> (w568:path)
                n418 = call "incNoStepsAcq.vi"("finPos"=w561, "initPos"=w542, "inp inc (mm)"=w560) -> ("no steps"=w533:i32, "out inc (mm)"=w540:dbl)
                n419 = call "incNoStepsAcq.vi"("finPos"=w559, "initPos"=w541, "inp inc (mm)"=w560) -> ("no steps"=w532:i32, "out inc (mm)"=w539:dbl)
                n420 = local write "z inc (mm)"(w555) -> ()
                n421 = Array Size(array=w534) -> (size(s)=w530:i32)
                n422 = local read "Filter wheel"() -> (w562:cluster{"FW Handle":u32, "init?":i16})
                n423 = local read "XY stage"() -> (w543:T3)
                n424 = local read "sCMOS"() -> (w566:cluster{"init":i16, "sCMOS handle":u32})
                n425 = local read "Z stage"() -> (w567:T2)
                n426 = call "createFilenameArray_slim.vi"("no x steps"=w533, "no y steps"=w532, "no z steps"=w531, "No colours"=w530, "Base path"=w568) -> ("stackFnameArray"=w538:path[][][], "frameFilenameArray"=w537:path[][][][])
              }
              frame #1 {
                n427 = Unbundle By Name(w611) -> ("sCMOS handle"=w610:u32)
                n428 = Unbundle By Name(w606) -> ("FW Handle"=w605:u32)
                n429 = Unbundle By Name(w616) -> ("System no."=w615:i32, "zIdx"=w614:i32)
                n430 = Unbundle By Name(w600) -> ("System no."=w599:i32, "xIdx"=w598:i32, "yIdx"=w597:i32)
                n431 = local read "coarse axial vel (mm/s)"() -> (w613:dbl)
                n432 = local read "acquisitionMode"() -> (w590:enum32{"stop/start  ", "cont."})
                n433 = local read "acqDelay (ms)"() -> (w612:u32)
                n434 = for {
                  tunnel: w619 -> [w672]
                  tunnel: w617 -> [w670]
                  shift-right: [w666] -> _
                  shift-left: w618 -> [w671]
                  tunnel: w607 -> [w662]
                  tunnel: w610 -> [w660]
                  tunnel: w592 -> [w658] mode=indexing
                  tunnel: w615 -> [w655]
                  tunnel: w614 -> [w654]
                  tunnel: w608 -> [w656]
                  tunnel: w609 -> [w651]
                  tunnel: w613 -> [w650]
                  tunnel: w590 -> [w649]
                  tunnel: w587 -> [w648]
                  tunnel: w612 -> [w647]
                  tunnel: w605 -> [w646]
                  tunnel: w604 -> [w645] mode=indexing
                  tunnel: w603 -> [w644] mode=indexing
                  tunnel: w602 -> [w643] mode=indexing
                  tunnel: w601 -> [w640] mode=indexing
                  tunnel: w599 -> [w637]
                  tunnel: w598 -> [w636]
                  tunnel: w597 -> [w635]
                  tunnel: w596 -> [w634]
                  tunnel: w595 -> [w633]
                  tunnel: w594 -> [w628]
                  tunnel: w593 -> [w621]
                  tunnel: [FALSE ("Acquisition in progress")] -> w588
                  stop <- w667 stop-if-true
                  n435 = Wait on Notification(notifier=w672, timeout in ms (-1)=w670, error in (no error)=w671) -> (timed out?=w668:bool, error out=w666:errorcluster)  [unwired: 1 in, 2 out]
                  n436 = flat-sequence {
                    tunnel: w670 -> [w694]
                    tunnel: w671 -> [w695]
                    tunnel: w672 -> [w696]
                    tunnel: [w696] -> w665
                    tunnel: [w695] -> w664
                    tunnel: [w694] -> w663
                    tunnel: w662 -> [w693]
                    tunnel: [w693] -> w661
                    tunnel: w660 -> [w692]
                    tunnel: [w692] -> w659
                    tunnel: w658 -> [w691]
                    tunnel: [w691] -> w657
                    tunnel: w656 -> [w687]
                    tunnel: w655 -> [w690]
                    tunnel: w654 -> [w689]
                    tunnel: [w688] -> w653
                    tunnel: [w687] -> w652
                    tunnel: w646 -> [w686]
                    tunnel: w645 -> [w685]
                    tunnel: w644 -> [w683]
                    tunnel: w643 -> [w684]
                    tunnel: [w683] -> w641
                    tunnel: w640 -> [w682]
                    tunnel: [w682] -> w638
                    tunnel: w637 -> [w677]
                    tunnel: w637 -> [w673]
                    tunnel: w636 -> [w676]
                    tunnel: w635 -> [w674]
                    tunnel: w634 -> [w675]
                    tunnel: w633 -> [w681]
                    tunnel: [w680] -> w632
                    tunnel: [w679] -> w631
                    tunnel: [w676] -> w630
                    tunnel: [w677] -> w629
                    tunnel: w628 -> [w678]
                    tunnel: [w678] -> w627
                    tunnel: [w677] -> w626
                    tunnel: [w676] -> w625
                    tunnel: [w675] -> w624
                    tunnel: [w674] -> w623
                    tunnel: [w673] -> w622
                    tunnel: w665 -> [w721]
                    tunnel: w664 -> [w720]
                    tunnel: w663 -> [w719]
                    tunnel: w661 -> [w718]
                    tunnel: w659 -> [w717]
                    tunnel: w657 -> [w716]
                    tunnel: w655 -> [w715]
                    tunnel: w654 -> [w714]
                    tunnel: w653 -> [_]
                    tunnel: w652 -> [w713]
                    tunnel: w651 -> [w712]
                    tunnel: w650 -> [w711]
                    tunnel: w649 -> [w710]
                    tunnel: w648 -> [w709]
                    tunnel: w647 -> [w708]
                    tunnel: [w707] -> w642
                    tunnel: w641 -> [w707]
                    tunnel: [w706] -> w639
                    tunnel: w638 -> [w706]
                    tunnel: w632 -> [_]
                    tunnel: w631 -> [_]
                    tunnel: w630 -> [w705]
                    tunnel: w629 -> [w704]
                    tunnel: w627 -> [w703]
                    tunnel: w626 -> [w702]
                    tunnel: w625 -> [w701]
                    tunnel: w624 -> [w700]
                    tunnel: w623 -> [w699]
                    tunnel: w622 -> [w698]
                    tunnel: w621 -> [w697]
                    tunnel: w642 -> [w875]
                    tunnel: w639 -> [w874]
                    frame #0 {
                      n437 = call "changeFWposAcq.vi"("FW pos"=w685, "FWhandle"=w686) -> ()
                      n438 = call "writeToSerialAcq.vi"("Cmmd"=w684, "input COM Port"=w683) -> ()
                      n439 = call "moveStageABS.vi"("absolute pos (mm)"=w687, "axisIdx"=w689, "System no."=w690) -> ("Stopped"=w688:bool)
                      n440 = call "moveStageABS.vi"("absolute pos (mm)"=w675, "axisIdx"=w676, "System no."=w677) -> ("Stopped"=w680:bool)
                      n441 = call "moveStageABS.vi"("absolute pos (mm)"=w681, "axisIdx"=w674, "System no."=w673) -> ("Stopped"=w679:bool)
                    }
                    frame #1 {
                      n442 = for {
                        tunnel: w721 -> [w750]
                        tunnel: w719 -> [w749]
                        shift-right: [w747] -> _
                        shift-left: w720 -> [w748]
                        tunnel: w718 -> [w743]
                        tunnel: w717 -> [w742]
                        tunnel: w716 -> [w741] mode=indexing
                        tunnel: w715 -> [w740]
                        tunnel: w714 -> [w739]
                        tunnel: w715 -> [w738]
                        tunnel: w714 -> [w737]
                        tunnel: w713 -> [w736]
                        tunnel: w712 -> [w735]
                        tunnel: w711 -> [w734]
                        tunnel: w710 -> [w733]
                        tunnel: w709 -> [w732]
                        tunnel: w708 -> [w731]
                        tunnel: w705 -> [w730]
                        tunnel: w704 -> [w729]
                        tunnel: w703 -> [w728]
                        tunnel: w702 -> [w727]
                        tunnel: w701 -> [w726]
                        tunnel: w700 -> [w725]
                        tunnel: w699 -> [w724]
                        tunnel: w698 -> [w723]
                        tunnel: w697 -> [w722]
                        stop <- w744 stop-if-true
                        n443 = Wait on Notification(notifier=w750, timeout in ms (-1)=w749, error in (no error)=w748) -> (timed out?=w746:bool, error out=w747:errorcluster)  [unwired: 1 in, 2 out]
                        n444 = flat-sequence {
                          tunnel: w750 -> [w769]
                          tunnel: w749 -> [w768]
                          tunnel: w748 -> [w767]
                          tunnel: w743 -> [w766]
                          tunnel: w742 -> [w765]
                          tunnel: w741 -> [w764]
                          tunnel: w740 -> [w763]
                          tunnel: w739 -> [w762]
                          tunnel: w738 -> [w761]
                          tunnel: w737 -> [w760]
                          tunnel: w736 -> [w759]
                          tunnel: w735 -> [w758]
                          tunnel: w734 -> [w757]
                          tunnel: w733 -> [w756]
                          tunnel: w732 -> [w755]
                          tunnel: w731 -> [w754]
                          tunnel: w730 -> [w753]
                          tunnel: w729 -> [w752]
                          tunnel: w728 -> [w751]
                          tunnel: [w873] -> _
                          tunnel: [w872] -> _
                          tunnel: w727 -> [w871]
                          tunnel: w726 -> [w870]
                          tunnel: w725 -> [w869]
                          tunnel: w724 -> [w868]
                          tunnel: w723 -> [w867]
                          tunnel: w722 -> [w866]
                          frame #0 {
                            n445 = for {
                              tunnel: w769 -> [w807]
                              shift-right: [w802] -> _
                              shift-left: w767 -> [w805]
                              tunnel: w768 -> [w806]
                              tunnel: w766 -> [w800]
                              tunnel: w765 -> [w788]
                              tunnel: w764 -> [w799] mode=indexing
                              tunnel: w763 -> [w798]
                              tunnel: w762 -> [w797]
                              tunnel: w761 -> [w796]
                              tunnel: w760 -> [w795]
                              tunnel: w759 -> [w794]
                              tunnel: w758 -> [w793]
                              tunnel: w757 -> [w792]
                              tunnel: w756 -> [w791]
                              tunnel: w755 -> [w790]
                              tunnel: w754 -> [w789]
                              tunnel: w753 -> [w787]
                              tunnel: w752 -> [w786]
                              tunnel: w751 -> [w785]
                              stop <- w801 stop-if-true
                              n446 = Wait on Notification(notifier=w807, timeout in ms (-1)=w806, error in (no error)=w805) -> (timed out?=w803:bool, error out=w802:errorcluster)  [unwired: 1 in, 2 out]
                              n447 = flat-sequence {
                                tunnel: w788 -> [w809]
                                tunnel: w789 -> [w810]
                                tunnel: w790 -> [w811]
                                tunnel: w791 -> [w812]
                                tunnel: w792 -> [w813]
                                tunnel: w793 -> [w814]
                                tunnel: w797 -> [w815]
                                tunnel: w798 -> [w816]
                                tunnel: w799 -> [w817]
                                tunnel: w800 -> [w818]
                                tunnel: w805 -> [w819]
                                tunnel: w806 -> [w820]
                                tunnel: w807 -> [w821]
                                tunnel: [w821] -> w784
                                tunnel: [w820] -> w783
                                tunnel: [w819] -> w782
                                tunnel: [w818] -> w781
                                tunnel: [w817] -> w780
                                tunnel: [w816] -> w779
                                tunnel: [w815] -> w778
                                tunnel: [w814] -> w777
                                tunnel: [w813] -> w776
                                tunnel: [w812] -> w775
                                tunnel: [w811] -> w774
                                tunnel: [w810] -> w773
                                tunnel: [w809] -> w772
                                tunnel: [w808] -> w771
                                tunnel: w784 -> [w835]
                                tunnel: w783 -> [w834]
                                tunnel: w782 -> [w833]
                                tunnel: w781 -> [w832]
                                tunnel: w780 -> [w831]
                                tunnel: w779 -> [w830]
                                tunnel: w778 -> [w829]
                                tunnel: w777 -> [w828]
                                tunnel: w776 -> [w827]
                                tunnel: w775 -> [w826]
                                tunnel: w774 -> [w825]
                                tunnel: w773 -> [w824]
                                tunnel: w772 -> [w823]
                                tunnel: w771 -> [w822]
                                tunnel: [w822] -> w770
                                tunnel: w796 -> [w865]
                                tunnel: w795 -> [w864]
                                tunnel: w794 -> [w863]
                                tunnel: [w862] -> _
                                tunnel: w787 -> [w861]
                                tunnel: w786 -> [w860]
                                tunnel: w785 -> [w859]
                                tunnel: [w858] -> _
                                tunnel: w770 -> [w856]
                                frame #0 {
                                n448 = Tick Count (ms)() -> (millisecond timer value=w808:u32)
                                }
                                frame #1 {
                                n449 = case shown="\"cont.\"" w826 {
                                tunnel: w835 -> [_ w849]
                                tunnel: w834 -> [_ w847]
                                tunnel: w833 -> [_ w848]
                                tunnel: w832 -> [_ w850]
                                tunnel: w831 -> [w844 w853]
                                tunnel: w830 -> [w839 w852]
                                tunnel: w829 -> [w838 w851]
                                tunnel: w828 -> [w836 _]
                                tunnel: w827 -> [w843 _]
                                tunnel: w825 -> [w837 _]
                                tunnel: w824 -> [w842 _]
                                tunnel: w823 -> [w840 w846]
                                tunnel: [w845 w854] -> _
                                frame "cont." {
                                n450 = call "contMotionAcq.vi"("sCMOS handle"=w840, "fine axial vel (mm/s)"=w836, "coarse axial vel (mm/s)"=w843, "System no."=w839, "zIdx"=w838, "z2"=w837, "imgFilenames"=w844, "stageAccDelay (ms)"="stageAccDelay (ms)", "acqDelay (ms)"=w842) -> ("Controller error"=w845:bool)  [unwired: 6 in]
                                }
                                frame "stop/start  ", Default {
                                n451 = call "stopStartMotionAcq.vi"("error out"=w848, "timeout"=w847, "notifier out"=w849, "frameFilenameArray"=w853, "z inc (mm)"=w850, "zIdx"=w851, "System no."=w852, "sCMOShandle"=w846) -> ("Stopped"=w854:bool)  [unwired: 2 in]
                                }
                                }
                                }
                                frame #2 {
                                n452 = call "moveStageABS.vi"("absolute pos (mm)"=w863, "axisIdx"=w864, "System no."=w865) -> ("Stopped"=w858:bool)
                                n453 = call "moveStage.vi"("inc (mm)"=w859, "axisIdx"=w861, "System no."=w860) -> ("Stopped"=w862:bool)
                                n454 = Tick Count (ms)() -> (millisecond timer value=w857:u32)
                                n455 = Subtract(x=w857, y=w856) -> (x-y=→"acquisitionTime":u32)
                                }
                              }
                              n456 = Unbundle By Name(w802) -> ("status"=w804:bool)
                              n457 = Compound Arithmetic op=OR(invert w803, w804) -> (w801:bool)
                            }
                          }
                          frame #1 {
                            n458 = call "moveStage.vi"("inc (mm)"=w866, "axisIdx"=w868, "System no."=w867) -> ("Stopped"=w873:bool)
                            n459 = call "moveStageABS.vi"("absolute pos (mm)"=w869, "axisIdx"=w870, "System no."=w871) -> ("Stopped"=w872:bool)
                          }
                        }
                        n460 = Unbundle By Name(w747) -> ("status"=w745:bool)
                        n461 = Compound Arithmetic op=OR(invert w746, w745) -> (w744:bool)
                      }
                    }
                    frame #2 {
                      n462 = call "writeToSerialAcq.vi"("Cmmd"=w874, "input COM Port"=w875) -> ()
                    }
                  }
                  n463 = Unbundle By Name(w666) -> ("status"=w669:bool)
                  n464 = Compound Arithmetic op=OR(invert w668, w669) -> (w667:bool)
                }
                "Acquisition in progress" <- w589
              }
              frame #2 {
                n465 = local write "Acquisition in progress"(w879) -> ()
                n466 = case shown="True" "convertDcimgToTifStacks" {
                  tunnel: w877 -> [_ w880]
                  tunnel: w876 -> [_ w881]
                  frame False {
                  }
                  frame True {
                    n467 = flat-sequence {
                      tunnel: [w885] -> w882
                      tunnel: w881 -> [w884]
                      tunnel: w880 -> [w883]
                      tunnel: w882 -> [w887]
                      frame #0 {
                        n468 = call "generateTiffStacks.vi"("singleImgFname"=w884, "stackFname"=w883) -> ("stackGenerationComplete"=w885:bool)
                        n469 = local write "Generating tiff stacks"(TRUE ("Generating tiff stacks")) -> ()
                      }
                      frame #1 {
                        "Generating tiff stacks" <- w887
                      }
                    }
                  }
                }
              }
            }
          }
          frame "idle", Default {
          }
          frame "mainStop" {
            # "Stutdown process here."
          }
          frame "cam1_live" {
            w899 = 1 items=["Snap", "Sequence"] ("Capture mode")
            n470 = local read "sCMOS"() -> (w902:cluster{"init":i16, "sCMOS handle":u32})
            n471 = Unbundle By Name(w902) -> ("sCMOS handle"=w898:u32)
            n472 = call <userlib>:"tm_preparecapture.vi"("Capture mode"=w899, "Handle in"=w898) -> ("error out"=w900:errorcluster, "Buffer Info"=w897:T8, "Handle out"=w901:u32)  [unwired: 6 in, 1 out]
            n473 = call <userlib>:"tm_startcapture_b.vi"("error in (no error)"=w900, "Handle in"=w901) -> ("error out"=w895:errorcluster, "Handle out"=w896:u32)  [unwired: 8 in]
            n474 = while {
              tunnel: w897 -> [w912]
              tunnel: w896 -> [w911]
              tunnel: w895 -> [w910]
              tunnel: w894 -> [w918]
              shift-right: [w916] -> _
              shift-left: w893 -> [w917]
              tunnel: [w907] -> w890
              tunnel: [w906] -> w889
              stop <- w905 stop-if-true
              n475 = call <userlib>:"tm_waitnextframe.vi"("error in (no error)"=w910, "Handle in"=w911) -> ("error out"=w913:errorcluster, "Frame Index"=w915:i32, "Handle out"=w914:u32)  [unwired: 6 in, 1 out]
              n476 = call <userlib>:"tm_getframe_a.vi"("error in (no error)"=w913, "Frame Index"=w915, "Buffer Info"=w912, "Handle in"=w914) -> ("error out"=w906:errorcluster, "Data 16"=w908:u16[][], "Handle out"=w907:u32)  [unwired: 3 in, 2 out]
              n477 = Wait on Notification(notifier=w918, timeout in ms (-1)=100, error in (no error)=w917) -> (timed out?=w920:bool, error out=w916:errorcluster)  [unwired: 1 in, 2 out]
              n478 = local read "stop live view"() -> (w903:bool)
              n479 = case shown="True" "View stream" {
                tunnel: w908 -> [_ w927]
                frame False {
                }
                frame True {
                  n480 = call "liveCameraView.vi"("Data 16"=w927) -> ("VI Refnum"=w925:refnum<vi>)
                  n481 = invoke class="VI" method="FP.Open"(reference=w925, "Activate"=FALSE ("Activate?"), "State"=T7."Standard") -> ()  [unwired: 2 in, 5 out]
                }
              }
              n482 = Unbundle By Name(w916) -> ("status"=w919:bool)
              n483 = Compound Arithmetic op=OR(invert w920, w919, "stop live stream", w903) -> (w905:bool)
              n484 = case shown="False" w905 {
                frame False {
                }
                frame True {
                  n485 = local write "Acquiring?"(FALSE ("Acquiring?")) -> ()
                }
              }
              "Acquiring?" <- TRUE ("Acquiring?")
            }
            n486 = call <userlib>:"tm_stopcapture.vi"("error in (no error)"=w889, "Handle in"=w890) -> ("error out"=w891:errorcluster, "Handle out"=w892:u32)  [unwired: 8 in]
            n487 = call <userlib>:"tm_unpreparecapture.vi"("error in (no error)"=w891, "Handle in"=w892) -> ()  [unwired: 8 in, 2 out]
          }
        }
      }
      frame Error {
        # "Return true in any case that should stop the loop."
      }
    }
  }
  n488 = Release Queue(queue=w23, error in (no error)=w27) -> (error out=w26:errorcluster)  [unwired: 1 in, 2 out]
  n489 = Release Notifier(notifier=w24, error in (no error)=w26) -> (error out=w25:errorcluster)  [unwired: 1 in, 2 out]
  n490 = call <vilib>:"General Error Handler.vi"("error in (no error)"=w25) -> ()  [unwired: 10 in, 5 out]
